vi "Auto - 副本.vi"() -> ()   [LabVIEW 2020]
uses:
  <vilib>/Utility/miscctls.llb/LVRowAndColumnTypeDef.ctl
  Global_Variable/A131258.vi
  Global_Variable/Global.vi
  Database/Global1.vi
  <vilib>/addons/database/Connection.llb/DB Tools Open Connec (String).vi
  <vilib>/addons/database/Connection.llb/Conn Execute.vi
  <vilib>/addons/database/Recordset.llb/Rec Fetch Recordset Data (R).vi
  Libraries/S7/S7.lvlib
  <vilib>/addons/database/NI_Database_API.lvlib
panel:
  out "左工位":cluster{dbl[], dbl[]}[](graph)
  in  "判定结果 2":bool[][](array[boolean])=[[TRUE]]
  out "STEP 4":string
  out "STEP 3":string
  in  "STEP 2":string
  out "右code 2":string
  in  "Initialize 7":bool
  in  "Initialize 6":bool
  out "初始化 2":bool[](array[boolean])
  out "左code":string
  out "右工位":cluster{dbl[], dbl[]}[](graph)
  in  "Initialize 4":bool
  in  "Initialize 2":bool
  out "初始化":bool[](array[boolean])
  in  "判定结果":bool[][](array[boolean])=[[TRUE]]
  in  "STEP":string
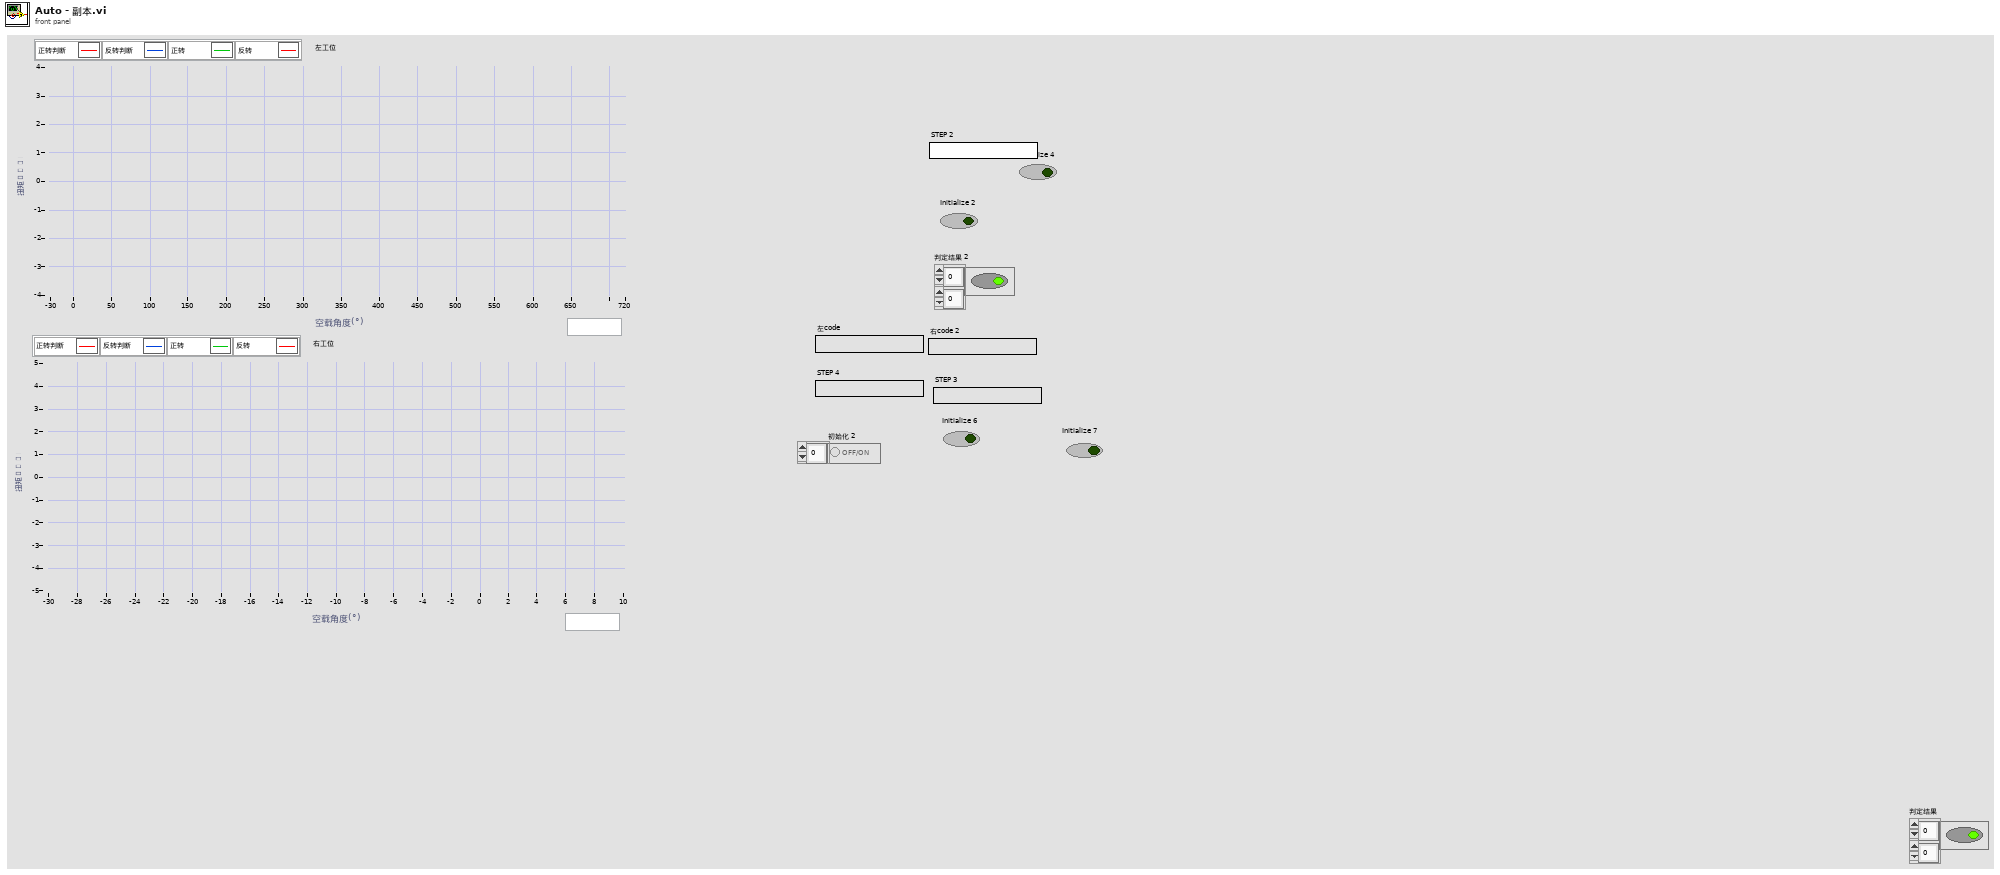
[diagram p1: front panel]
types:
  T1 = enum32{"Invalid", "Standard", "Closed", "Hidden", "Minimized", "Maximized"}
  T2 = typedef "LVRowAndColumnTypeDef.ctl" = cluster{"Row":i32, "Column":i32}
  T3 = typedef "lveventtype.ctl" = enum32{"Null", "Timeout", "Annotation Menu Selection", "Annotation Menu Selection?", "App Instance Close", "App Instance Close?", "Autoscale Range Change", "Bookmark Info Change", "Cell Edit", "Cell Edit?", "Cursor Grab", "Cursor Grab?", "Cursor Menu Selection", "Cursor Menu Selection?", "Cursor Move", "Cursor Release", "Data Change", "Direction Change", "Display State Change", "Drag Ended", "Drag Enter", "Drag Leave", "Drag Over", "Drag Source Update", "Drag Starting", "Drag Starting?", "Drop", "Exec State Change", "Key Down", "Key Down?", "Key Repeat", "Key Repeat?", "Key Up", "Listbox Double Click", "Menu Activation?", "Menu Selection (App)", "Menu Selection? (App)", "Menu Selection (User)", "Mouse Down", "Mouse Down?", "Mouse Enter", "Mouse Leave", "Mouse Move", "Mouse Up", "Mouse Wheel", "NI Security User Change (App)", "Pane Size", "Panel Close", "Panel Close?", "Panel Resize", "Plot Attribute Change", "Scale Range Change", "Shortcut Menu Activation?", "Shortcut Menu Selection (App)", "Shortcut Menu Selection? (App)", "Shortcut Menu Selection (User)", "Tree Double Click", "Tree Drag", "Tree Drag?", "Tree Drop", "Tree Drop?", "Tree Item Close", "Tree Item Close?", "Tree Item Open", "Tree Item Open?", "User Event", "Value Change"}
  T4 = typedef "LVPoint32TypeDef.ctl" = cluster{"Horizontal":i32, "Vertical":i32}
  T5 = cluster{"扭矩判定":cluster{"单位":string, "下限":dbl, "上限":dbl}, "正转扭矩最大值":cluster{"单位":string, "下限":dbl, "上限":dbl}, "正转扭矩最小值":cluster{"单位":string, "下限":dbl, "上限":dbl}, "正转扭矩波动值":cluster{"单位":string, "下限":dbl, "上限":dbl}, "正转平均扭矩值":cluster{"单位":string, "下限":dbl, "上限":dbl}, "反转扭矩最大值":cluster{"单位":string, "下限":dbl, "上限":dbl}, "反转扭矩最小值":cluster{"单位":string, "下限":dbl, "上限":dbl}, "反转扭矩波动值":cluster{"单位":string, "下限":dbl, "上限":dbl}, "反转扭矩平均值":cluster{"单位":string, "下限":dbl, "上限":dbl}, "正/逆转平均扭矩差":cluster{"单位":string, "下限":dbl, "上限":dbl}}
  T6 = cluster{"正向判定X值":cluster{"单位":string, "下限":dbl, "上限":dbl}, "正向判定Y值":cluster{"单位":string, "下限":dbl, "上限":dbl}, "逆向判定X值":cluster{"单位":string, "下限":dbl, "上限":dbl}, "逆向判定Y值":cluster{"单位":string, "下限":dbl, "上限":dbl}}
  T7 = cluster{"左平均扭矩":cluster{"正转":dbl, "反转":dbl}, "左矩波动":cluster{"正转":dbl, "反转":dbl}, "左空载":cluster{"正转":dbl, "反转":dbl}, "右平均扭矩":cluster{"正转":dbl, "反转":dbl}, "右扭矩波动":cluster{"正转":dbl, "反转":dbl}, "右空载":cluster{"正转":dbl, "反转":dbl}, "扭矩对称":cluster{"左":dbl, "右":dbl}, "左零点漂移":cluster{"正":dbl, "反":dbl}, "右零点漂移":cluster{"正":dbl, "反":dbl}}
  T8 = typedef "NI_Database_API.lvlib/Conn ObjectReference.ctl" = refnum<k1>
  T9 = typedef "NI_Database_API.lvlib/Rec ObjectReference.ctl" = refnum<k1>
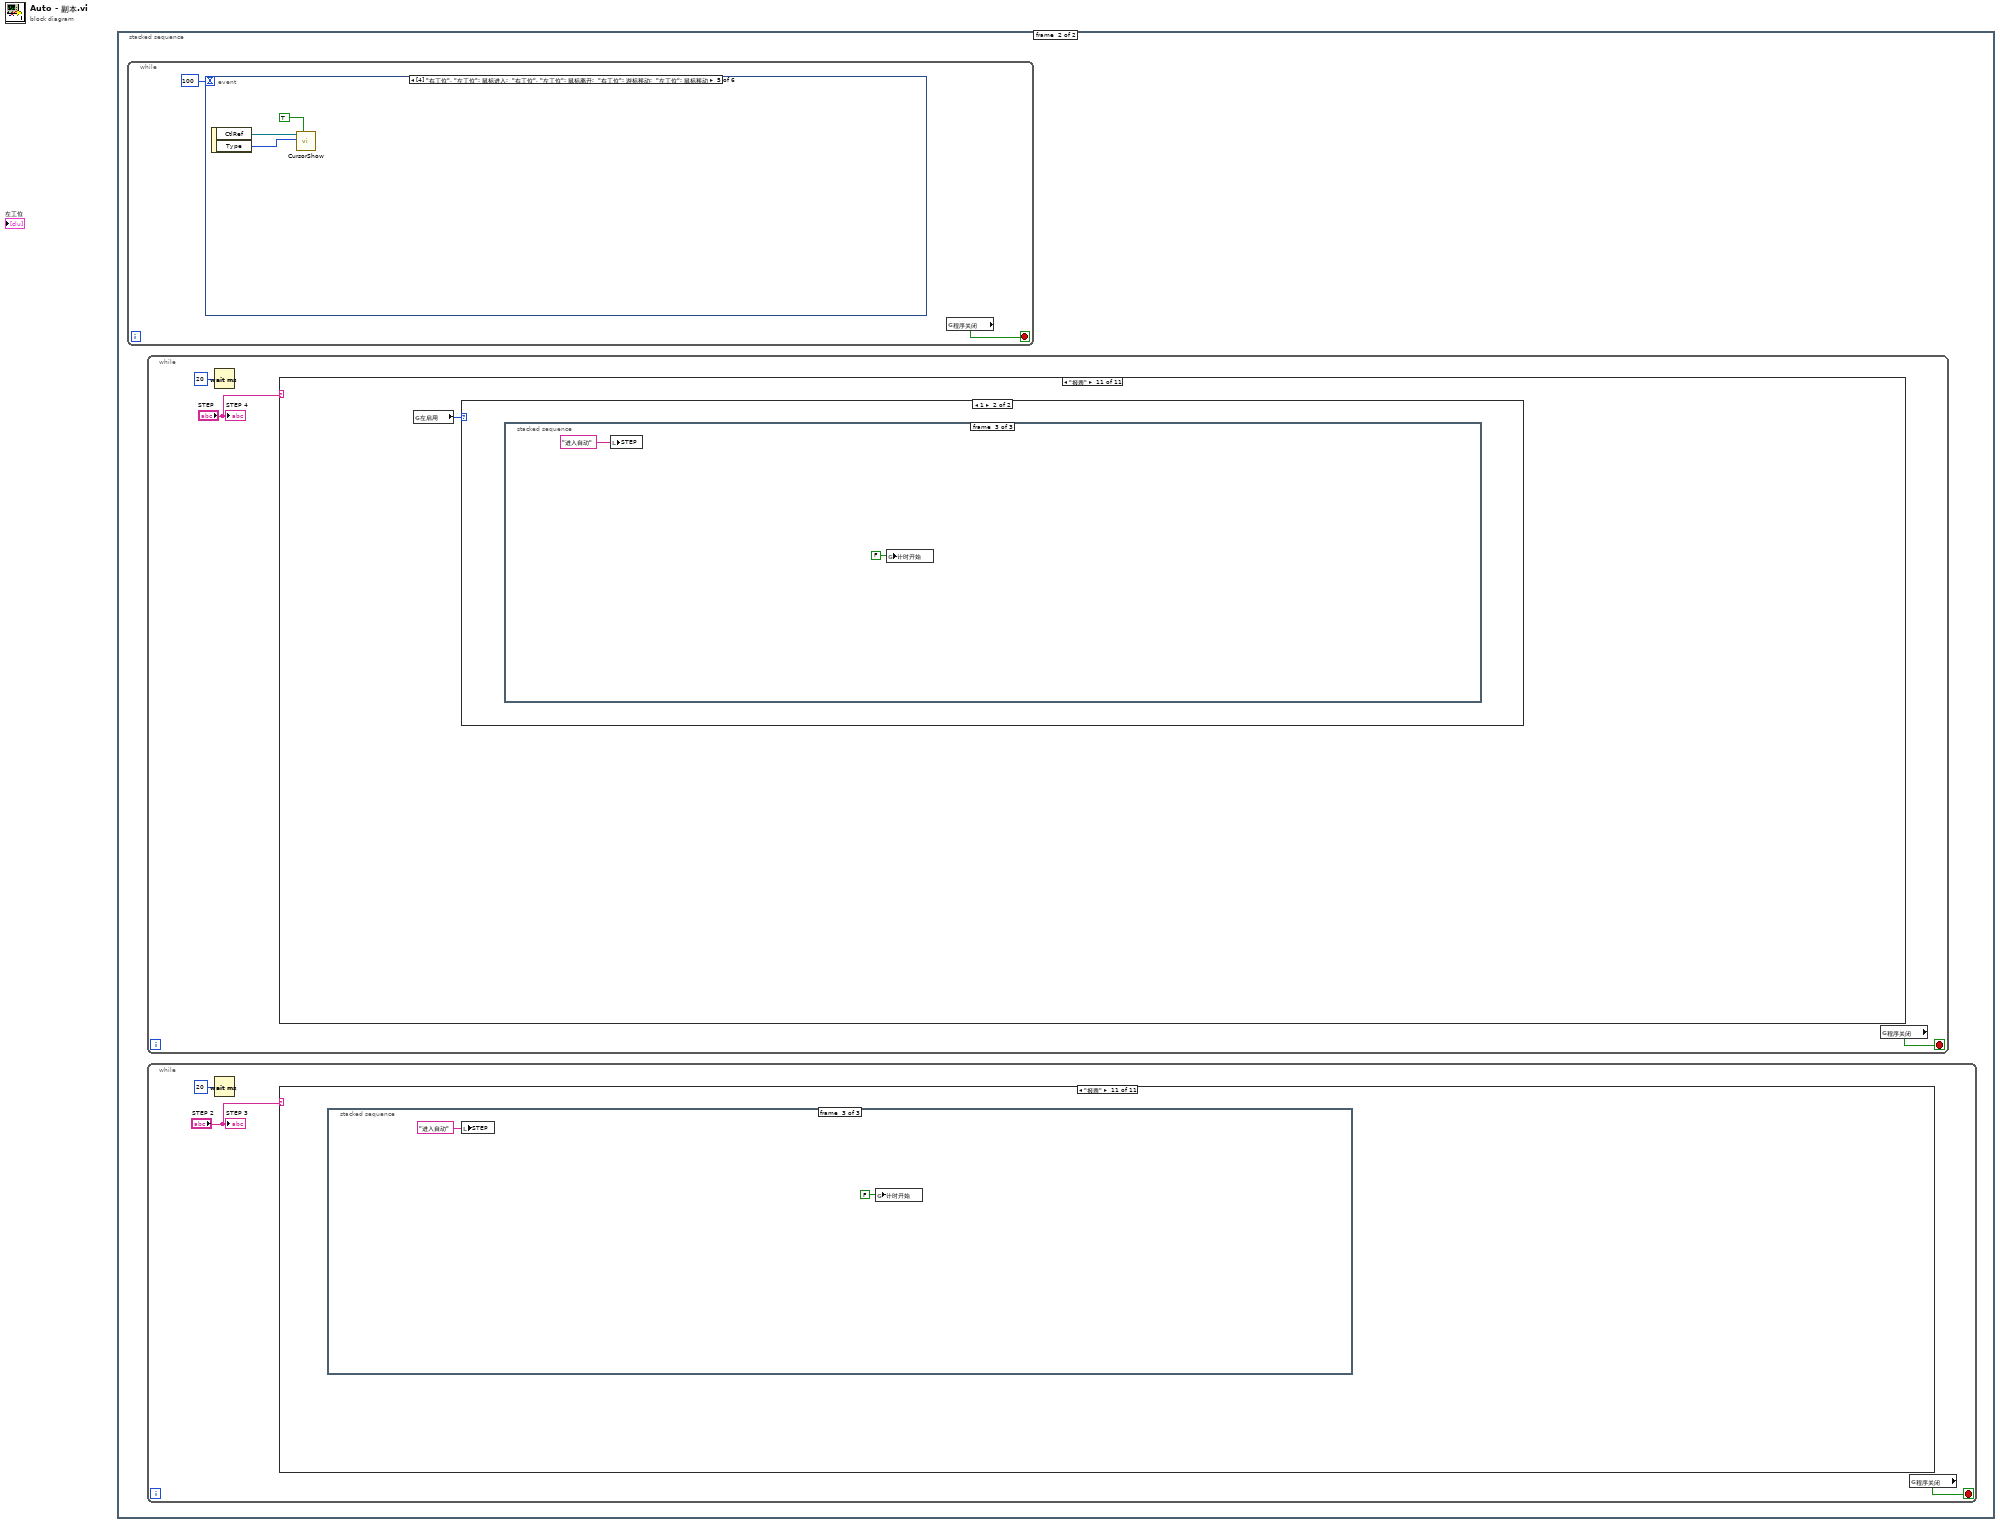
[diagram p0: block diagram]
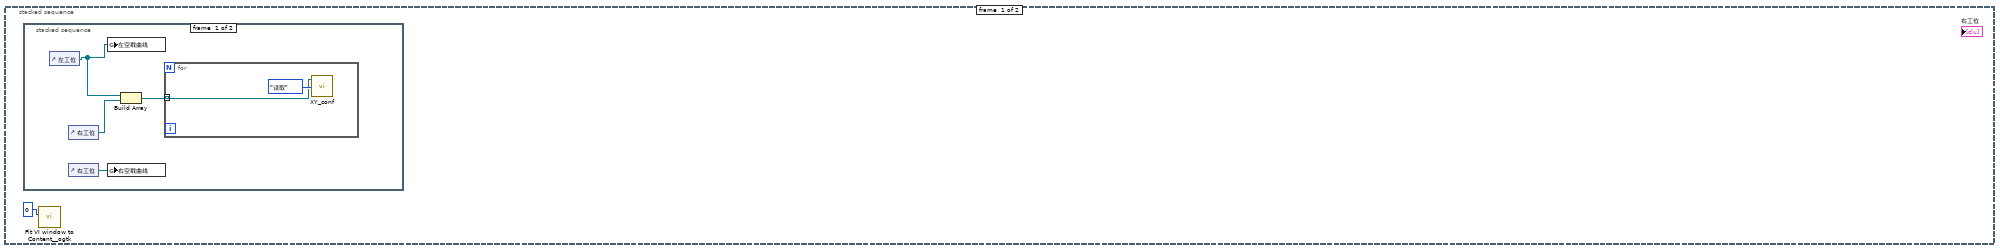
[diagram p2: hidden frame]
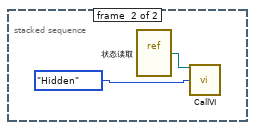
[diagram p3: hidden frame]
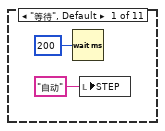
[diagram p4: hidden frame]
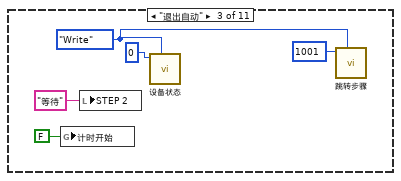
[diagram p6: hidden frame]
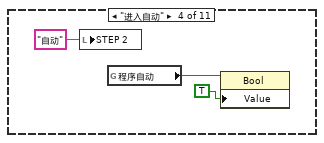
[diagram p7: hidden frame]
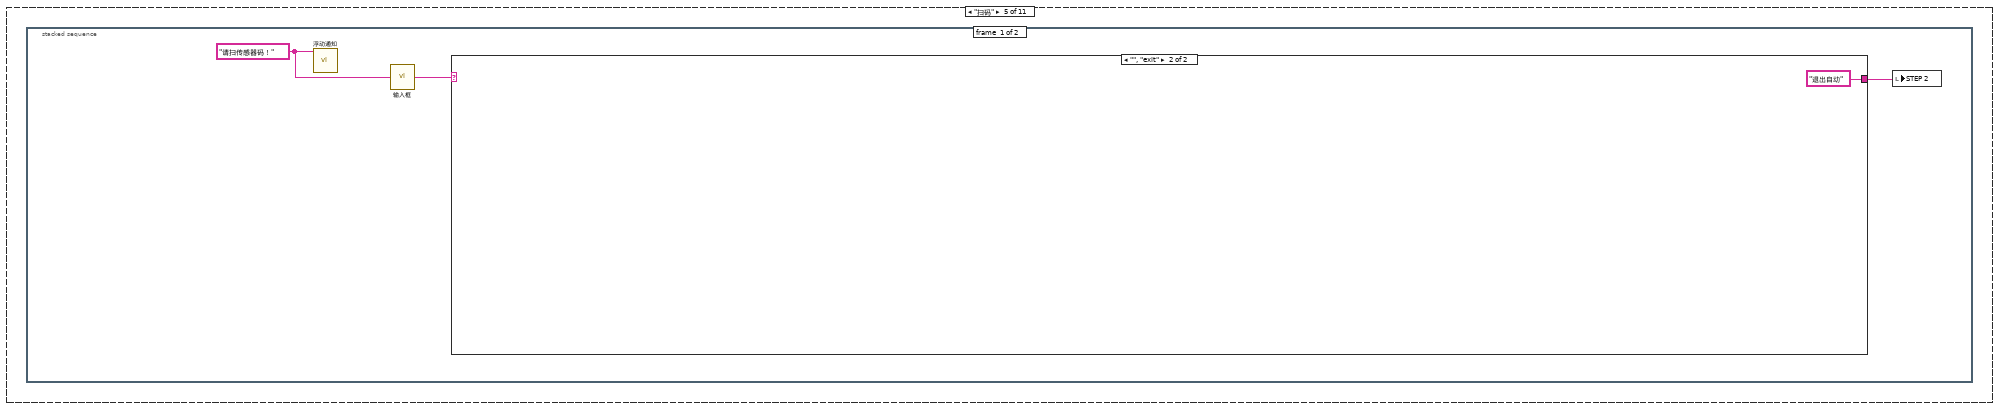
[diagram p8: hidden frame]
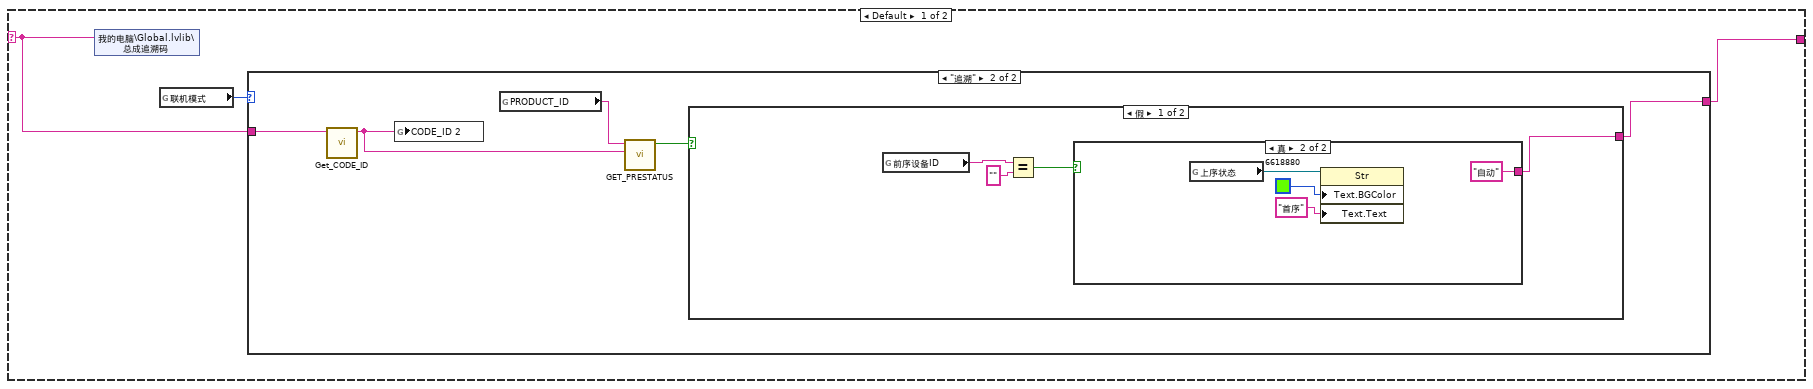
[diagram p9: hidden frame]
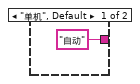
[diagram p10: hidden frame]
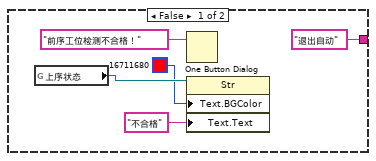
[diagram p11: hidden frame]
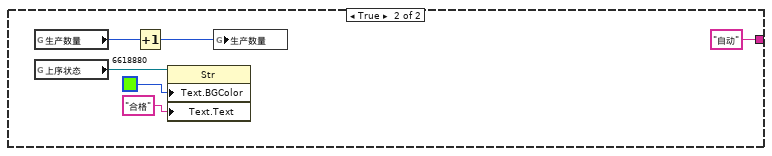
[diagram p12: hidden frame]
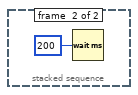
[diagram p13: hidden frame]
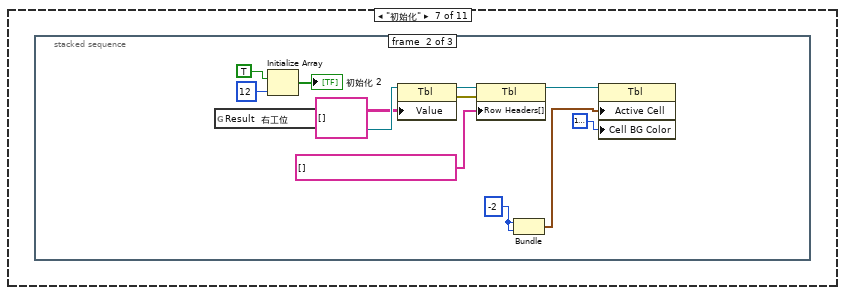
[diagram p15: hidden frame]
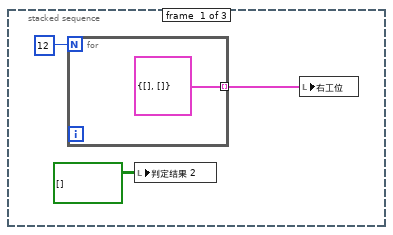
[diagram p16: hidden frame]
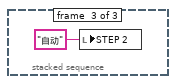
[diagram p17: hidden frame]
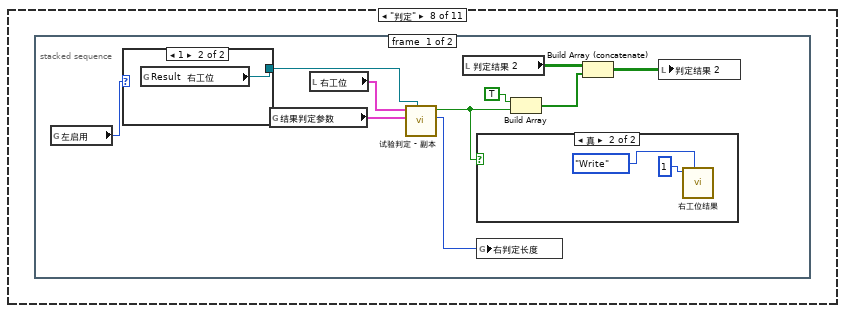
[diagram p18: hidden frame]
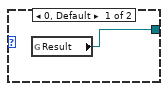
[diagram p19: hidden frame]
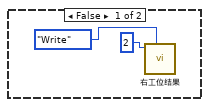
[diagram p20: hidden frame]
diagram:
  n1 = stacked-sequence {
    frame #0 {
      n2 = stacked-sequence {
        frame #0 {
          n3 = control-ref of="左工位"() -> (w2:refnum<vi>)
          n4 = control-ref of="右工位"() -> (w4:refnum<vi>)
          n5 = control-ref of="右工位"() -> (w5:refnum<vi>)
          n6 = global write "A131258.vi" "左空载曲线"(w2) -> ()
          n7 = global write "A131258.vi" "右空载曲线"(w5) -> ()
          n8 = Build Array(w2, w4) -> (w3:refnum<vi>[])
          n9 = for {
            tunnel: w3 -> [w6] mode=indexing
            n10 = call "XY_conf.vi"("方式"=enum16{"写入", "读取"}."读取", "XY图引用"=w6) -> ()  [unwired: 3 in, 1 out]
          }
        }
        frame #1 {
          n11 = vi-ref "状态读取.vi"() -> (w9:refnum<vi>)
          n12 = call "CallVI.vi"("VI引用"=w9, "状态"=T1."Hidden") -> ()  [unwired: 11 in, 3 out]
        }
      }
      n13 = call <userlib>:"Fit VI window to Content__ogtk.vi"("border spacing (2 px)"=0) -> ()  [unwired: 5 in, 2 out]
    }
    frame #1 {
      n14 = while {
        stop <- w748 stop-if-true
        n15 = event shown="[4] \"右工位\", \"左工位\": 鼠标进入;  \"右工位\", \"左工位\": 鼠标离开;  \"右工位\": 游标移动;  \"左工位\": 鼠标移动" {
          selector: _ -> [_ _ _ _ _ _]
          dyn-events: _ -> [_ _ _ _ _ _]
          timeout: 100 -> [_ _ _ _ _ _]
          event Timeout {
            n16 = event-data() -> ()  [unwired: 1 in, 3 out]
            n17 = call "Obtain Broadcast Events for Registration.vi"() -> ("Already running?"=w750:bool)  [unwired: 9 in, 2 out]
            n18 = case shown="真" w750 {
              frame False {
                n19 = local write "STEP"("手动" ("STEP")) -> ()
              }
              frame True {
                n20 = call "错误代码.vi"() -> ("Status_Read"=w752:u32)  [unwired: 11 in]
                n21 = case shown="0" w752 {
                  frame 0 {
                    n22 = global read "Global.vi" "报警图标"() -> (w763:refnum<vi>)
                    n23 = property class="Bool"(reference=w763, "Visible"=FALSE ("可见")) -> ()  [unwired: 1 in, 2 out]
                  }
                  frame 1, Default {
                    n24 = global read "Global.vi" "报警图标"() -> (w766:refnum<vi>)
                    n25 = property class="Bool"(reference=w766, "Visible"=TRUE ("可见")) -> ()  [unwired: 1 in, 2 out]
                  }
                }
                n26 = feedback #1() -> (w762:u32)  [unwired: 1 in]
                n27 = feedback-in #1(w752) -> ()
                n28 = Greater Or Equal?(x=w752, y=i16 5000) -> (x >= y?=w760:bool)
                n29 = Less?(x=w752, y=i16 5200) -> (x < y?=w761:bool)
                n30 = Equal?(x=w752, y=w762) -> (x = y?=w759:bool)
                n31 = global read "Global.vi" "报警图标"() -> (w754:refnum<vi>)
                n32 = And(x=w760, y=w761) -> (x .and. y?=w753:bool)
                n33 = property class="Bool"(reference=w754, "Value"=w753) -> ()  [unwired: 1 in, 2 out]
                n34 = Bundle By Name(cluster=errorcluster {"status"=FALSE, "code"=0, "source"=""} ("错误常量"), "status"=w753, "code"=w752) -> (w758:errorcluster)
                n35 = case shown="假" w759 {
                  tunnel: w758 -> [w767 _]
                  frame False {
                    n36 = call "报警处理.vi"("错误常量"=w767) -> ()  [unwired: 9 in, 2 out]
                  }
                  frame True {
                  }
                }
              }
            }
          }
          event Menu Selection (User) {
            n37 = event-data() -> ("ItemTag"=w768:string)  [unwired: 1 in, 2 out]
            n38 = case shown="\"真\"" w768 {
              frame "假", Default {
              }
              frame "真" {
              }
            }
          }
          event "右工位", "左工位": Scale Range Change {
            n39 = event-data() -> ("CtlRef"=w769:refnum<vi>)  [unwired: 1 in]
            n40 = call "XY_conf.vi"("方式"=enum16{"写入", "读取"}."写入", "XY图引用"=w769) -> ()  [unwired: 3 in, 1 out]
          }
          event Panel Close {
            n41 = event-data() -> ()  [unwired: 1 in, 4 out]
            n42 = global write "Global.vi" "程序关闭"(TRUE ("程序关闭")) -> ()
          }
          event "右工位", "左工位": Mouse Enter; "右工位", "左工位": Mouse Leave; "右工位": Cursor Move; "左工位": Mouse Move {
            n43 = event-data() -> ("CtlRef"=w774:refnum<vi>, "Type"=w773:T3)  [unwired: 1 in]
            n44 = call "CursorShow.vi"("nameShow"=TRUE, "Type"=w773, "Graph"=w774) -> ()  [unwired: 7 in, 2 out]
          }
          event "右工位", "左工位": Mouse Down {
            n45 = event-data() -> ("CtlRef"=w779:refnum<vi>, "Coords"=w778:T4, "Type"=w777:T3)  [unwired: 1 in]
            n46 = invoke class="XYGraph (严格)" method="Map Coords To XY"(reference=w779, "Coords"=w778) -> (reference out=w776:refnum<vi>, "XY"=w775:cluster{"X":dbl, "Y":dbl})  [unwired: 5 in, 5 out]
            n47 = call "CursorShow.vi"("游标.游标位置"=w775, "Type"=w777, "Graph"=w776) -> ()  [unwired: 7 in, 2 out]
          }
        }
        n48 = global read "Global.vi" "程序关闭"() -> (w748:bool)
      }
      n49 = while {
        stop <- w374 stop-if-true
        n50 = Wait (ms)(milliseconds to wait=u32 20 ("等待时间（毫秒）")) -> ()  [unwired: 1 out]
        n51 = case shown="\"报表\"" "STEP" {
          frame "等待", Default {
            n52 = Wait (ms)(milliseconds to wait=u32 200 ("等待时间（毫秒）")) -> ()  [unwired: 1 out]
            n53 = local write "STEP"("自动" ("STEP")) -> ()
          }
          frame "手动" {
          }
          frame "退出自动" {
            w378 = enum16{"Read", "Write"}."Write" ("枚举")
            n54 = global write "Global.vi" "计时开始"(FALSE ("计时开始")) -> ()
            n55 = local write "STEP"("等待" ("STEP")) -> ()
            n56 = call "设备状态.vi"("枚举"=w378, "Status_Write"=i16 0) -> ()  [unwired: 9 in, 1 out]
            n57 = call "跳转步骤.vi"("枚举"=w378, "Status_Write"=i16 1001) -> ()  [unwired: 9 in, 1 out]
          }
          frame "进入自动" {
            n58 = local write "STEP"("自动" ("STEP")) -> ()
            n59 = global read "Global.vi" "程序自动"() -> (w383:refnum<vi>)
            n60 = property class="Bool"(reference=w383, "Value"=TRUE) -> ()  [unwired: 1 in, 2 out]
          }
          frame "扫码" {
            n61 = stacked-sequence {
              frame #0 {
                w386 = "请扫传感器码！" ("提示信息")
                n62 = call "浮动通知.vi"("通知内容"=w386) -> ()  [unwired: 11 in]
                n63 = call "输入框.vi"("提示信息"=w386) -> ("条形码输出"=w387:string)
                n64 = case shown="\"\", \"exit\"" w387 {
                  selector: w387 -> [w388 _]
                  tunnel: [w390 "退出自动" ("State(s) in Front (\"\")")] -> w385
                  frame Default {
                    n65 = shared-variable "我的电脑\\Global.lvlib\\工位追溯码"(w388) -> ()  [unwired: 1 in, 1 out]
                    n66 = global read "Global1.vi" "联机模式"() -> (w389:enum16{"单机", "追溯"})
                    n67 = case shown="\"追溯\"" w389 {
                      tunnel: ["自动" ("State(s) in Front (\"\")") w396] -> w390
                      tunnel: w388 -> [_ w395]
                      frame "单机", Default {
                      }
                      frame "追溯" {
                        n68 = call "Get_CODE_ID.vi"("CODE_MAIN"=w395) -> ("CODE_ID"=w392:string)  [unwired: 10 in]
                        n69 = global write "追溯Global.vi" "CODE_ID"(w392) -> ()
                        n70 = global read "追溯Global.vi" "PRODUCT_ID"() -> (w394:string)
                        n71 = call "GET_PRESTATUS.vi"("CODE_ID"=w392, "PRODUCT_ID"=w394) -> ("OK?"=w393:bool)  [unwired: 8 in, 1 out]
                        n72 = case shown="真" w393 {
                          tunnel: [w400 "自动" ("State(s) in Front (\"\")")] -> w396
                          frame False {
                            n73 = global read "追溯Global.vi" "前序设备ID"() -> (w399:string)
                            n74 = Equal?(x=w399, y="") -> (x = y?=w398:bool)
                            n75 = case shown="真" w398 {
                              tunnel: ["退出自动" ("State(s) in Front (\"\")") "自动" ("State(s) in Front (\"\")")] -> w400
                              frame False {
                                n76 = global read "Global.vi" "上序状态"() -> (w403:refnum<vi>)
                                n77 = One Button Dialog(message="前序工位检测不合格！" ("消息")) -> ()  [unwired: 1 in, 1 out]
                                n78 = property class="Str"(reference=w403, "Text.BGColor"=u32 16711680 ("文本.文本颜色:背景色"), "Text.Text"="不合格" ("文本.文本")) -> ()  [unwired: 1 in, 2 out]
                              }
                              frame True {
                                n79 = global read "Global.vi" "上序状态"() -> (w408:refnum<vi>)
                                n80 = property class="Str"(reference=w408, "Text.BGColor"=u32 6618880 ("文本.文本颜色:背景色"), "Text.Text"="首序" ("文本.文本")) -> ()  [unwired: 1 in, 2 out]
                              }
                            }
                          }
                          frame True {
                            n81 = global read "Global.vi" "生产数量"() -> (w413:i32)
                            n82 = global read "Global.vi" "上序状态"() -> (w412:refnum<vi>)
                            n83 = Increment(x=w413) -> (x+1=w414:i32)
                            n84 = property class="Str"(reference=w412, "Text.BGColor"=u32 6618880 ("文本.文本颜色:背景色"), "Text.Text"="合格" ("文本.文本")) -> ()  [unwired: 1 in, 2 out]
                            n85 = global write "Global.vi" "生产数量"(w414) -> ()
                          }
                        }
                      }
                    }
                  }
                  frame "", "exit" {
                  }
                }
                n86 = local write "STEP"(w385) -> ()
              }
              frame #1 {
                n87 = Wait (ms)(milliseconds to wait=u32 200 ("等待时间（毫秒）")) -> ()  [unwired: 1 out]
              }
            }
          }
          frame "工位判断" {
          }
          frame "初始化" {
            n88 = stacked-sequence {
              frame #0 {
                n89 = global write "Global.vi" "IO_Stop"(TRUE ("IO_Stop")) -> ()
                n90 = global write "Global.vi" "计时开始"(TRUE ("计时开始")) -> ()
                n91 = local write "判定结果"(bool[][] [] ("判定结果")) -> ()
              }
              frame #1 {
                n92 = for {
                  N: 12 -> [_]
                  tunnel: [cluster{dbl[], dbl[]} {[], []}] -> w421 mode=indexing
                }
                n93 = local write "左工位"(w421) -> ()
              }
              frame #2 {
                w424 = -2 ("维数大小")
                n94 = global read "Global.vi" "Result"() -> (w433:refnum<vi>)
                n95 = Initialize Array(TRUE, 12 ("维数大小")) -> (→"初始化":bool[])
                n96 = property class="Tbl"(reference=w433, "Value"=string[][] []) -> (reference out=w434:refnum<vi>, error out=w435:errorcluster)  [unwired: 1 in]
                n97 = property class="Tbl"(reference=w434, error in=w435, "Row Headers[]"=string[] [] ("列首字符串[]")) -> (reference out=w427:refnum<vi>)  [unwired: 1 out]
                n98 = Bundle("维数大小"=w424, "维数大小"=w424) -> (w425:cluster{"维数大小":i32, "维数大小":i32})  [unwired: 1 in]
                n99 = property class="Tbl"(reference=w427, "Active Cell"=w425, "Cell BG Color"=u32 16777216 ("活动单元格:单元格背景色")) -> ()  [unwired: 1 in, 2 out]
              }
              frame #3 {
                n100 = local write "STEP"("自动" ("STEP")) -> ()
              }
            }
          }
          frame "判定" {
            n101 = stacked-sequence {
              frame #0 {
                n102 = global read "A131258.vi" "结果判定参数"() -> (w438:T5)
                n103 = global read "Global.vi" "Result"() -> (w440:refnum<vi>)
                n104 = local read "左工位"() -> (w439:cluster{dbl[], dbl[]}[])
                n105 = call "试验判定.vi"("Result"=w440, "判定参数"=w438, "XY曲线"=w439) -> ("判定项长度"=w437:i32, "OK？"=w441:bool)  [unwired: 7 in]
                n106 = case shown="真" w441 {
                  frame False {
                    n107 = call "左工位结果.vi"("枚举"=enum16{"Read", "Write"}."Write", "Status_Write"=u16 2 ("左工位生产结果")) -> ()  [unwired: 9 in, 1 out]
                  }
                  frame True {
                    n108 = call "左工位结果.vi"("枚举"=enum16{"Read", "Write"}."Write", "Status_Write"=u16 1 ("左工位生产结果")) -> ()  [unwired: 9 in, 1 out]
                  }
                }
                n109 = global write "判定参数.vi" "左判定长度"(w437) -> ()
                n110 = Build Array(TRUE ("元素"), w441) -> (w444:bool[])
                n111 = local read "判定结果"() -> (w445:bool[][])
                n112 = Build Array(w444) -> (w443:bool[][])
                n113 = Build Array (concatenate)(w445, w443) -> (w446:bool[][])
                n114 = local write "判定结果"(w446) -> ()
              }
              frame #1 {
                n115 = local write "STEP"("报表" ("STEP")) -> ()
              }
            }
          }
          frame "自动" {
            n116 = global read "Global.vi" "跳转"() -> (w452:i16)
            n117 = global read "Global.vi" "左状态"() -> (w453:i16)
            n118 = case shown="1003" w452 {
              frame 0, Default {
              }
              frame 1000 {
                n119 = stacked-sequence {
                  frame #0 {
                    w454 = "" ("文本.文本")
                    n120 = Wait (ms)(milliseconds to wait=u32 200 ("等待时间（毫秒）")) -> ()  [unwired: 1 out]
                    n121 = shared-variable "我的电脑\\Global.lvlib\\传感器码-左"(w454) -> ()  [unwired: 1 in, 1 out]
                    n122 = shared-variable "我的电脑\\Global.lvlib\\传感器码-右"(w454) -> ()  [unwired: 1 in, 1 out]
                    n123 = call "跳转步骤.vi"("枚举"=enum16{"Read", "Write"}."Write", "Status_Write"=u16 1001 ("跳转步骤")) -> ()  [unwired: 9 in, 1 out]
                  }
                  frame #1 {
                    n124 = local write "STEP"("扫码" ("STEP")) -> ()
                  }
                }
              }
              frame 1001 {
                n125 = stacked-sequence {
                  frame #0 {
                    n126 = Wait (ms)(milliseconds to wait=u32 100 ("等待时间（毫秒）")) -> ()  [unwired: 1 out]
                  }
                  frame #1 {
                    n127 = global read "Global.vi" "左在位"() -> (w461:i16)
                    n128 = global read "Global.vi" "右在位"() -> (w460:i16)
                    n129 = case shown="1" w461 {
                      frame 0, Default {
                      }
                      frame 1 {
                        w466 = enum16{"Read", "Write"}."Write" ("枚举")
                        n130 = call "左工位在位.vi"("枚举"=w466, "Status_Write"=u16 0 ("左工位工件在位")) -> ()  [unwired: 9 in, 1 out]
                        n131 = call "左工位状态.vi"("枚举"=w466, "Status_Write"=u16 1001 ("左工位状态")) -> ()  [unwired: 9 in, 1 out]
                      }
                    }
                    n132 = case shown="1" w460 {
                      frame 0, Default {
                      }
                      frame 1 {
                        w462 = enum16{"Read", "Write"}."Write" ("枚举")
                        n133 = call "右工位在位.vi"("枚举"=w462, "Status_Write"=u16 0 ("右工位工件在位")) -> ()  [unwired: 9 in, 1 out]
                        n134 = call "右工位状态.vi"("枚举"=w462, "Status_Write"=u16 1001 ("左工位状态")) -> ()  [unwired: 9 in, 1 out]
                      }
                    }
                  }
                  frame #2 {
                    n135 = local write "STEP 2"("自动" ("STEP")) -> ()
                    n136 = local write "STEP"("自动" ("STEP")) -> ()
                  }
                }
              }
              frame 1002 {
                # "SELECT CODE_ID FROM CODE  WHERE CODE_SENSOR = '"
                n137 = stacked-sequence {
                  frame #0 {
                    n138 = Wait (ms)(milliseconds to wait=u32 200 ("等待时间（毫秒）")) -> ()  [unwired: 1 out]
                    n139 = call "跳转步骤.vi"("枚举"=enum16{"Read", "Write"}."Write", "Status_Write"=u16 1003 ("跳转步骤")) -> ()  [unwired: 9 in, 1 out]
                  }
                  frame #1 {
                    n140 = local write "STEP 2"("扫码" ("STEP")) -> ()
                  }
                }
              }
              frame 1003 {
                n141 = stacked-sequence {
                  frame #0 {
                    n142 = Wait (ms)(milliseconds to wait=u32 100 ("等待时间（毫秒）")) -> ()  [unwired: 1 out]
                  }
                  frame #1 {
                    n143 = global read "Global.vi" "左在位"() -> (w476:i16)
                    n144 = global read "Global.vi" "右在位"() -> (w475:i16)
                    n145 = case shown="1" w476 {
                      frame 0, Default {
                      }
                      frame 1 {
                        w480 = enum16{"Read", "Write"}."Write" ("枚举")
                        n146 = call "左工位在位.vi"("枚举"=w480, "Status_Write"=u16 0 ("左工位工件在位")) -> ()  [unwired: 9 in, 1 out]
                        n147 = call "左工位状态.vi"("枚举"=w480, "Status_Write"=u16 1002 ("左工位状态")) -> ()  [unwired: 9 in, 1 out]
                      }
                    }
                    n148 = case shown="1" w475 {
                      frame 0, Default {
                      }
                      frame 1 {
                        w477 = enum16{"Read", "Write"}."Write" ("枚举")
                        n149 = call "右工位在位.vi"("枚举"=w477, "Status_Write"=u16 0 ("右工位工件在位")) -> ()  [unwired: 9 in, 1 out]
                        n150 = call "右工位状态.vi"("枚举"=w477, "Status_Write"=u16 1002 ("左工位状态")) -> ()  [unwired: 9 in, 1 out]
                      }
                    }
                  }
                  frame #2 {
                    w483 = "自动" ("STEP")
                    n151 = local write "STEP"(w483) -> ()
                    n152 = local write "STEP 2"(w483) -> ()
                  }
                }
              }
            }
            n153 = case shown="1002" w453 {
              frame 0, Default {
              }
              frame 1 {
              }
              frame 3 {
                n154 = stacked-sequence {
                  frame #0 {
                    n155 = call "左工位结果.vi"("枚举"=enum16{"Read", "Write"}."Write", "Status_Write"=i16 0) -> ()  [unwired: 9 in, 1 out]
                    n156 = local write "判定结果"(bool[][] [] ("判定结果")) -> ()
                  }
                  frame #1 {
                    n157 = global read "Global.vi" "空载速度(°/s) 2"() -> (w487:sgl)
                    n158 = Multiply(x=w487, y=sgl 6.0) -> (x*y=w488:sgl)
                    n159 = global write "Global.vi" "空载速度(°/s)"(w488) -> ()
                  }
                }
              }
              frame 200 {
                n160 = stacked-sequence {
                  frame #0 {
                    w490 = TRUE ("Initialize 2")
                    n161 = local write "Initialize 2"(w490) -> ()
                    n162 = local write "Initialize 4"(w490) -> ()
                    n163 = call "左工位结果.vi"("枚举"=enum16{"Read", "Write"}."Write", "Status_Write"=u16 0 ("左工位生产结果")) -> ()  [unwired: 9 in, 1 out]
                  }
                  frame #1 {
                    n164 = local read "左工位"() -> (w493:cluster{dbl[], dbl[]}[])
                    n165 = for {
                      tunnel: [w496] -> w494 mode=indexing
                      tunnel: w493 -> [w495] mode=indexing
                      i -> [w497]
                      n166 = case shown="1" w497 {
                        tunnel: [w498 w499 w507] -> w496
                        tunnel: w495 -> [w498 _ _]
                        frame Default {
                        }
                        frame 0 {
                          n167 = global read "A131258.vi" "判定框参数"() -> (w504:T6)
                          n168 = Unbundle By Name(w504) -> ("正向判定X值.下限"=w503:dbl, "正向判定X值.上限"=w502:dbl, "正向判定Y值.下限"=w501:dbl, "正向判定Y值.上限"=w500:dbl)
                          n169 = Build Array(w502, w502, w503, w503, w502) -> (w506:dbl[])
                          n170 = Build Array(w500, w501, w501, w500, w500) -> (w505:dbl[])
                          n171 = Bundle(w506, w505) -> (w499:cluster{dbl[], dbl[]})  [unwired: 1 in]
                        }
                        frame 1 {
                          n172 = global read "A131258.vi" "判定框参数"() -> (w512:T6)
                          n173 = Unbundle By Name(w512) -> ("逆向判定X值.下限"=w511:dbl, "逆向判定X值.上限"=w510:dbl, "逆向判定Y值.下限"=w509:dbl, "逆向判定Y值.上限"=w508:dbl)
                          n174 = Build Array(w510, w510, w511, w511, w510) -> (w514:dbl[])
                          n175 = Build Array(w508, w509, w509, w508, w508) -> (w513:dbl[])
                          n176 = Bundle(w514, w513) -> (w507:cluster{dbl[], dbl[]})  [unwired: 1 in]
                        }
                      }
                    }
                    n177 = local write "左工位"(w494) -> ()
                  }
                }
              }
              frame 500 {
                n178 = local read "左工位"() -> (w516:cluster{dbl[], dbl[]}[])
                n179 = for {
                  tunnel: w516 -> [w518] mode=indexing
                  tunnel: [w517] -> w515 mode=indexing
                  i -> [w519]
                  n180 = case shown="2" w519 {
                    tunnel: w518 -> [w520 w537]
                    tunnel: [w520 w528] -> w517
                    frame Default {
                    }
                    frame 2 {
                      n181 = local write "Initialize 2"(FALSE ("Initialize 2")) -> ()
                      n182 = global read "A131258.vi" "系数"() -> (w523:T7)
                      n183 = case shown="假" "Initialize 2" {
                        tunnel: [w550 0.0] -> w533
                        frame False {
                          n184 = global read "全局 1.vi" "工位2正向磨合开始时间"() -> (w554:u32)
                          n185 = Tick Count (ms)() -> (millisecond timer value=w553:u32)
                          n186 = Subtract(x=w553, y=w554) -> (x-y=w552:u32)
                          n187 = Divide(x=w552, y=u32 1000) -> (x/y=w550:dbl)
                          n188 = global write "全局 1.vi" "工位2正向磨合结束时间"(w550) -> ()
                        }
                        frame True {
                          n189 = Tick Count (ms)() -> (millisecond timer value=w555:u32)
                          n190 = global write "全局 1.vi" "工位2正向磨合开始时间"(w555) -> ()
                        }
                      }
                      n191 = global read "A131258.vi" "零点标定"() -> (w524:bool)
                      n192 = global read "全局1.vi" "左加载"() -> (w522:dbl)
                      n193 = case shown="假" w524 {
                        tunnel: [w539 w546] -> w521
                        tunnel: w523 -> [w545 w549]
                        tunnel: w522 -> [w544 w548]
                        frame False {
                          n194 = Unbundle By Name(w545) -> ("左零点漂移.正"=w543:dbl, "左空载.正转"=w540:dbl, "左零点漂移.正"=w538:dbl)
                          n195 = Multiply(x=w544, y=w543) -> (x*y=w541:dbl)
                          n196 = Subtract(x=w541, y=w540) -> (x-y=w542:dbl)
                          n197 = Subtract(x=w542, y=w538) -> (x-y=w539:dbl)
                        }
                        frame True {
                          n198 = Unbundle By Name(w549) -> ("左零点漂移.正"=w547:dbl)
                          n199 = Subtract(x=w548, y=w547) -> (x-y=w546:dbl)
                        }
                      }
                      n200 = Unbundle(w537) -> (w530:dbl[], w536:dbl[])
                      n201 = Build Array (concatenate)(w536, w521) -> (w527:dbl[])
                      n202 = global read "Global.vi" "空载速度(°/s)"() -> (w532:sgl)
                      n203 = Divide(x=w533, y=1.0) -> (x/y=w526:dbl)
                      n204 = Multiply(x=w532, y=w526) -> (x*y=w531:dbl)
                      n205 = Build Array (concatenate)(w530, w531) -> (w529:dbl[])
                      n206 = Bundle(w529, w527) -> (w528:cluster{dbl[], dbl[]})  [unwired: 1 in]
                    }
                  }
                }
                n207 = local write "左工位"(w515) -> ()
              }
              frame 600 {
                n208 = local read "左工位"() -> (w558:cluster{dbl[], dbl[]}[])
                n209 = for {
                  tunnel: w558 -> [w560] mode=indexing
                  tunnel: [w559] -> w557 mode=indexing
                  i -> [w561]
                  n210 = case shown="3" w561 {
                    tunnel: w560 -> [w562 w579]
                    tunnel: [w562 w570] -> w559
                    frame 0, Default {
                    }
                    frame 3 {
                      n211 = local write "Initialize 4"(FALSE ("Initialize 2")) -> ()
                      n212 = case shown="假" "Initialize 4" {
                        tunnel: [w592 w599] -> w576
                        frame False {
                          n213 = global read "全局 1.vi" "工位2逆向磨合开始时间"() -> (w598:u32)
                          n214 = Tick Count (ms)() -> (millisecond timer value=w597:u32)
                          n215 = Subtract(x=w597, y=w598) -> (x-y=w596:u32)
                          n216 = global read "全局 1.vi" "工位2正向磨合结束时间"() -> (w594:dbl)
                          n217 = Divide(x=w596, y=u32 1000) -> (x/y=w593:dbl)
                          n218 = Subtract(x=w594, y=w593) -> (x-y=w592:dbl)
                        }
                        frame True {
                          n219 = Tick Count (ms)() -> (millisecond timer value=w600:u32)
                          n220 = global write "全局 1.vi" "工位2逆向磨合开始时间"(w600) -> ()
                          n221 = global read "全局 1.vi" "工位2正向磨合结束时间"() -> (w599:dbl)
                        }
                      }
                      n222 = global read "全局1.vi" "左加载"() -> (w564:dbl)
                      n223 = global read "A131258.vi" "系数"() -> (w565:T7)
                      n224 = global read "A131258.vi" "零点标定"() -> (w566:bool)
                      n225 = Unbundle(w579) -> (w573:dbl[], w578:dbl[])
                      n226 = case shown="假" w566 {
                        tunnel: [w581 w588] -> w563
                        tunnel: w565 -> [w587 w591]
                        tunnel: w564 -> [w586 w590]
                        frame False {
                          n227 = Unbundle By Name(w587) -> ("左零点漂移.反"=w585:dbl, "左空载.反转"=w582:dbl, "左零点漂移.反"=w580:dbl)
                          n228 = Multiply(x=w586, y=w585) -> (x*y=w583:dbl)
                          n229 = Subtract(x=w583, y=w582) -> (x-y=w584:dbl)
                          n230 = Subtract(x=w584, y=w580) -> (x-y=w581:dbl)
                        }
                        frame True {
                          n231 = Unbundle By Name(w591) -> ("左零点漂移.反"=w589:dbl)
                          n232 = Add(x=w590, y=w589) -> (x+y=w588:dbl)
                        }
                      }
                      n233 = Build Array (concatenate)(w578, w563) -> (w571:dbl[])
                      n234 = global read "Global.vi" "空载速度(°/s)"() -> (w575:sgl)
                      n235 = Divide(x=w576, y=1.0) -> (x/y=w568:dbl)
                      n236 = Multiply(x=w575, y=w568) -> (x*y=w574:dbl)
                      n237 = Build Array (concatenate)(w573, w574) -> (w572:dbl[])
                      n238 = Bundle(w572, w571) -> (w570:cluster{dbl[], dbl[]})  [unwired: 1 in]
                    }
                  }
                }
                n239 = local write "左工位"(w557) -> ()
              }
              frame 680 {
                n240 = local write "STEP"("判定" ("STEP")) -> ()
              }
              frame 1001 {
                n241 = stacked-sequence {
                  frame #0 {
                    n242 = Wait (ms)(milliseconds to wait=u32 50 ("等待时间（毫秒）")) -> ()  [unwired: 1 out]
                    n243 = shared-variable "我的电脑\\Global.lvlib\\工位追溯码"() -> (w602:string)  [unwired: 1 in, 1 out]
                    n244 = shared-variable "我的电脑\\Global.lvlib\\传感器码-左"(w602) -> ()  [unwired: 1 in, 1 out]
                  }
                  frame #1 {
                    n245 = global read "Global1.vi" "联机模式"() -> (w604:enum16{"单机", "追溯"})
                    n246 = case shown="\"追溯\"" w604 {
                      selector: w604 -> [_ w614]
                      frame "单机", Default {
                      }
                      frame "追溯" {
                        n247 = shared-variable "我的电脑\\Global.lvlib\\传感器码-左"() -> (w605:string)  [unwired: 1 in, 1 out]
                        n248 = global read "追溯Global.vi" "PRODUCT_ID"() -> (w611:string)
                        n249 = Bundle("String"=w605, "PRODUCT_ID"=w611) -> (w610:cluster{"String":string, "PRODUCT_ID":string})  [unwired: 1 in]
                        n250 = call "GetSQLstring.vi"("联机模式"=w614) -> ("错误输出"=w612:errorcluster, "连接字符串"=w613:string)  [unwired: 9 in]
                        n251 = call-poly <vilib>:"DB Tools Open Connection.vi"("error in (no error)"=w612, "connection information"=w613) -> ("error out"=w608:errorcluster, "connection reference"=w609:T8)  [unwired: 6 in]
                        n252 = Build Array(w610) -> (w606:cluster{"String":string, "PRODUCT_ID":string}[])
                        n253 = for {
                          tunnel: w609 -> [w622]
                          shift-right: [w619] -> w607
                          shift-left: w608 -> [w621]
                          tunnel: w606 -> [w615] mode=indexing
                          n254 = call <vilib>:"DB Tools Insert Data.vi"("data"=w615, "error in (no error)"=w621, "columns"=string[] ["CODE_SENSOR", "PRODUCT_ID"], "table"="Code", "connection reference"=w622) -> ("error out"=w620:errorcluster, "connection reference out"=w618:T8)  [unwired: 5 in]
                          n255 = case shown="错误 .." w620 {
                            selector: w620 -> [w624 w626]
                            tunnel: [w624 w627] -> w619
                            tunnel: [w623 w625] -> _
                            tunnel: w618 -> [w623 w625]
                            frame No Error {
                            }
                            frame Error {
                              n256 = call <vilib>:"Clear Errors.vi"("error in (no error)"=w626) -> ("error out"=w627:errorcluster)  [unwired: 5 in, 1 out]
                            }
                          }
                        }
                        n257 = call <vilib>:"Simple Error Handler.vi"("error in (no error)"=w607) -> ()  [unwired: 4 in, 5 out]
                      }
                    }
                  }
                  frame #2 {
                    n258 = global read "Global1.vi" "联机模式"() -> (w628:enum16{"单机", "追溯"})
                    n259 = case shown="\"追溯\"" w628 {
                      selector: w628 -> [_ w649]
                      frame "单机", Default {
                      }
                      frame "追溯" {
                        w641 = "'"
                        n260 = shared-variable "我的电脑\\Global.lvlib\\传感器码-左"() -> (w629:string)  [unwired: 1 in, 1 out]
                        n261 = global read "追溯Global.vi" "PRODUCT_ID"() -> (w642:string)
                        n262 = call "GetSQLstring.vi"("联机模式"=w649) -> ("错误输出"=w647:errorcluster, "连接字符串"=w648:string)  [unwired: 9 in]
                        n263 = Concatenate Strings("SELECT CODE_ID FROM CODE  WHERE CODE_SENSOR = '" ("table"), w629, w641, " AND PRODUCT_ID='" ("字符串"), w642, w641) -> (w640:string)
                        n264 = call-poly <vilib>:"DB Tools Open Connection.vi"("error in (no error)"=w647, "connection information"=w648) -> ("error out"=w646:errorcluster, "connection reference"=w645:T8)  [unwired: 6 in]
                        n265 = call-poly <vilib>:"DB Tools Execute Query.vi"("error in (no error)"=w646, "SQL query"=w640, "connection reference"=w645) -> ("error out"=w639:errorcluster, "recordset reference"=w638:T9)  [unwired: 5 in]
                        n266 = call-poly <vilib>:"DB Tools Fetch Recordset Data.vi"("error in (no error)"=w639, "recordset reference"=w638) -> ("error out"=w637:errorcluster, "recordset data"=w636:variant[][])  [unwired: 3 in, 1 out]
                        n267 = Variant To Data(error in=w637, type=string[][] [], Variant=w636) -> (data=w634:string[][])  [unwired: 1 out]
                        n268 = Index Array(array=w634, index (row)=0 ("索引 (行)")) -> (element=w633:string[])  [unwired: 1 in]
                        n269 = Index Array(array=w633, index=0 ("索引")) -> (element=→"左code":string)
                      }
                    }
                  }
                  frame #3 {
                    n270 = Wait (ms)(milliseconds to wait=u32 50 ("等待时间（毫秒）")) -> ()  [unwired: 1 out]
                    n271 = call "左工位状态.vi"("枚举"=enum16{"Read", "Write"}."Write", "Status_Write"=u16 1003 ("左工位状态")) -> ()  [unwired: 9 in, 1 out]
                    n272 = for {
                      N: 12 -> [_]
                      tunnel: [cluster{dbl[], dbl[]} {[], []}] -> w656 mode=indexing
                    }
                    n273 = local write "左工位"(w656) -> ()
                    n274 = global read "Global.vi" "Result"() -> (w654:refnum<vi>)
                    n275 = property class="Tbl"(reference=w654, "Row Headers[]"=string[] [] ("行首字符串[]"), "Value"=string[][] [] ("值"), "Active Cell"=T2 {"Row"=-2, "Column"=-2} ("活动单元格:活动单元格"), "Cell BG Color"=u32 16777216 ("活动单元格:单元格背景色")) -> ()  [unwired: 1 in, 2 out]
                  }
                }
              }
              frame 1002 {
                n276 = stacked-sequence {
                  frame #0 {
                    n277 = Wait (ms)(milliseconds to wait=u32 100 ("等待时间（毫秒）")) -> ()  [unwired: 1 out]
                    n278 = shared-variable "我的电脑\\Global.lvlib\\总成追溯码"() -> (w661:string)  [unwired: 1 in, 1 out]
                    n279 = shared-variable "我的电脑\\Global.lvlib\\传感器码-左"(w661) -> ()  [unwired: 1 in, 1 out]
                  }
                  frame #1 {
                    n280 = global read "Global1.vi" "联机模式"() -> (w663:enum16{"单机", "追溯"})
                    n281 = case shown="\"追溯\"" w663 {
                      selector: w663 -> [_ w673]
                      frame "单机", Default {
                      }
                      frame "追溯" {
                        n282 = shared-variable "我的电脑\\Global.lvlib\\传感器码-左"() -> (w664:string)  [unwired: 1 in, 1 out]
                        n283 = global read "追溯Global.vi" "PRODUCT_ID"() -> (w672:string)
                        n284 = Bundle("String"=w664, "PRODUCT_ID"=w672) -> (w670:cluster{"String":string, "PRODUCT_ID":string})  [unwired: 1 in]
                        n285 = call "GetSQLstring.vi"("联机模式"=w673) -> ("错误输出"=w669:errorcluster, "连接字符串"=w671:string)  [unwired: 9 in]
                        n286 = call-poly <vilib>:"DB Tools Open Connection.vi"("error in (no error)"=w669, "connection information"=w671) -> ("error out"=w666:errorcluster, "connection reference"=w668:T8)  [unwired: 6 in]
                        n287 = Build Array(w670) -> (w665:cluster{"String":string, "PRODUCT_ID":string}[])
                        n288 = for {
                          tunnel: w665 -> [w680] mode=indexing
                          tunnel: w668 -> [w679]
                          shift-right: [w675] -> w667
                          shift-left: w666 -> [w674]
                          n289 = call <vilib>:"DB Tools Insert Data.vi"("data"=w680, "error in (no error)"=w674, "columns"=string[] ["CODE_SENSOR", "PRODUCT_ID"], "table"="Code", "connection reference"=w679) -> ("error out"=w676:errorcluster)  [unwired: 5 in, 1 out]
                          n290 = case shown="无错误" w676 {
                            selector: w676 -> [w681 w682]
                            tunnel: [w681 w683] -> w675
                            frame No Error {
                            }
                            frame Error {
                              n291 = call <vilib>:"Clear Errors.vi"("error in (no error)"=w682) -> ("error out"=w683:errorcluster)  [unwired: 5 in, 1 out]
                            }
                          }
                        }
                        n292 = call <vilib>:"Simple Error Handler.vi"("error in (no error)"=w667) -> ()  [unwired: 4 in, 5 out]
                      }
                    }
                  }
                  frame #2 {
                    n293 = global read "Global1.vi" "联机模式"() -> (w684:enum16{"单机", "追溯"})
                    n294 = case shown="\"追溯\"" w684 {
                      selector: w684 -> [_ w705]
                      frame "单机", Default {
                      }
                      frame "追溯" {
                        w697 = "'"
                        n295 = shared-variable "我的电脑\\Global.lvlib\\传感器码-左"() -> (w685:string)  [unwired: 1 in, 1 out]
                        n296 = global read "追溯Global.vi" "PRODUCT_ID"() -> (w698:string)
                        n297 = call "GetSQLstring.vi"("联机模式"=w705) -> ("错误输出"=w703:errorcluster, "连接字符串"=w704:string)  [unwired: 9 in]
                        n298 = Concatenate Strings("SELECT CODE_ID FROM CODE  WHERE CODE_SENSOR = '" ("table"), w685, w697, " AND PRODUCT_ID='" ("字符串"), w698, w697) -> (w696:string)
                        n299 = call-poly <vilib>:"DB Tools Open Connection.vi"("error in (no error)"=w703, "connection information"=w704) -> ("error out"=w702:errorcluster, "connection reference"=w701:T8)  [unwired: 6 in]
                        n300 = call-poly <vilib>:"DB Tools Execute Query.vi"("error in (no error)"=w702, "SQL query"=w696, "connection reference"=w701) -> ("error out"=w695:errorcluster, "recordset reference"=w694:T9)  [unwired: 5 in]
                        n301 = call-poly <vilib>:"DB Tools Fetch Recordset Data.vi"("error in (no error)"=w695, "recordset reference"=w694) -> ("error out"=w693:errorcluster, "recordset data"=w692:variant[][])  [unwired: 3 in, 1 out]
                        n302 = Variant To Data(error in=w693, type=string[][] [], Variant=w692) -> (data=w690:string[][])  [unwired: 1 out]
                        n303 = Index Array(array=w690, index (row)=0 ("索引 (行)")) -> (element=w689:string[])  [unwired: 1 in]
                        n304 = Index Array(array=w689, index=0 ("索引")) -> (element=w688:string)
                        n305 = local write "左code"(w688) -> ()
                      }
                    }
                  }
                  frame #3 {
                    n306 = local write "STEP"("自动" ("STEP")) -> ()
                    n307 = call "左工位状态.vi"("枚举"=enum16{"Read", "Write"}."Write", "Status_Write"=u16 1003 ("左工位状态")) -> ()  [unwired: 9 in, 1 out]
                    n308 = for {
                      N: 12 -> [_]
                      tunnel: [cluster{dbl[], dbl[]} {[], []}] -> w712 mode=indexing
                    }
                    n309 = local write "左工位"(w712) -> ()
                    n310 = global read "Global.vi" "Result"() -> (w711:refnum<vi>)
                    n311 = property class="Tbl"(reference=w711, "Row Headers[]"=string[] [] ("行首字符串[]"), "Value"=string[][] [] ("值"), "Active Cell"=T2 {"Row"=-2, "Column"=-2} ("活动单元格:活动单元格"), "Cell BG Color"=u32 16777216 ("活动单元格:单元格背景色")) -> ()  [unwired: 1 in, 2 out]
                  }
                }
              }
            }
          }
          frame "不合格" {
            n312 = Wait (ms)(milliseconds to wait=u32 100 ("等待时间（毫秒）")) -> ()  [unwired: 1 out]
            n313 = local write "STEP"("等待" ("STEP")) -> ()
          }
          frame "报表" {
            n314 = global read "Global.vi" "左启用"() -> (w719:i16)
            n315 = case shown="1" w719 {
              frame 0, Default {
              }
              frame 1 {
                n316 = stacked-sequence {
                  frame #0 {
                    n317 = stacked-sequence {
                      seq-local: [w722 _ _] -> [_ w725 _]
                      frame #0 {
                        n318 = shared-variable "我的电脑\\Global.lvlib\\传感器码-左"() -> (w720:string)  [unwired: 1 in, 1 out]
                        n319 = call "Report.vi"("文件重命名"=TRUE, "文件名称"=w720, "检测结果"="判定结果") -> ("PRODUCT_VAULE"=w722:string)  [unwired: 7 in, 1 out]
                      }
                      frame #1 {
                        n320 = global read "Global1.vi" "联机模式"() -> (w724:enum16{"单机", "追溯"})
                        n321 = case shown="\"追溯\"" w724 {
                          tunnel: w725 -> [_ w729]
                          frame "单机", Default {
                          }
                          frame "追溯" {
                            n322 = global read "Global.vi" "Result"() -> (w733:refnum<vi>)
                            n323 = property class="Tbl"(reference=w733) -> (reference out=w732:refnum<vi>, "Row Headers[]"=w730:string[])  [unwired: 1 in, 1 out]
                            n324 = property class="Tbl"(reference=w732) -> ("Value"=w731:string[][])  [unwired: 1 in, 2 out]
                            n325 = for {
                              tunnel: w731 -> [w737] mode=indexing
                              tunnel: w730 -> [w738] mode=indexing
                              tunnel: [w735] -> w727 mode=indexing if=w736
                              n326 = Build Array (concatenate)(w738, w737) -> (w735:string[])
                              n327 = Index Array(array=w737) -> (element=w739:string)  [unwired: 1 in]
                              n328 = case shown="\"\"" w739 {
                                tunnel: [TRUE FALSE] -> w736
                                frame Default {
                                }
                                frame "" {
                                }
                              }
                            }
                            n329 = global read "追溯Global.vi" "DEVICE_ID"() -> (w728:string)
                            n330 = global read "追溯Global.vi" "USER_ID"() -> (w734:string)
                            n331 = local read "左code"() -> (w726:string)
                            n332 = call "UPTEST.vi"("Result"=w727, "CODE_ID"=w726, "DEVICE_ID"=w728) -> ()  [unwired: 6 in, 1 out]
                            n333 = call "UPRESULT.vi"("DEVICE_ID"=w728, "USER_ID"=w734, "CODE_ID"=w726, "RESULT_VALUE"=w729) -> ()  [unwired: 11 in, 1 out]
                          }
                        }
                      }
                      frame #2 {
                        n334 = Wait (ms)(milliseconds to wait=u32 50 ("等待时间（毫秒）")) -> ()  [unwired: 1 out]
                      }
                    }
                  }
                  frame #1 {
                    n335 = global write "Global.vi" "计时开始"(FALSE ("计时开始")) -> ()
                    n336 = call "左工位状态.vi"("枚举"=enum16{"Read", "Write"}."Write", "Status_Write"=i16 3) -> ()  [unwired: 9 in, 1 out]
                  }
                  frame #2 {
                    n337 = local write "STEP"("进入自动" ("STEP")) -> ()
                    n338 = global write "Global.vi" "计时开始"(FALSE ("计时开始")) -> ()
                  }
                }
              }
            }
          }
        }
        n339 = global read "Global.vi" "程序关闭"() -> (w374:bool)
        "STEP 4" <- "STEP"
      }
      n340 = while {
        stop <- w12 stop-if-true
        n341 = Wait (ms)(milliseconds to wait=u32 20 ("等待时间（毫秒）")) -> ()  [unwired: 1 out]
        n342 = case shown="\"报表\"" "STEP 2" {
          frame "等待", Default {
            n343 = Wait (ms)(milliseconds to wait=u32 200 ("等待时间（毫秒）")) -> ()  [unwired: 1 out]
            n344 = local write "STEP"("自动" ("STEP")) -> ()
          }
          frame "手动" {
          }
          frame "退出自动" {
            w16 = enum16{"Read", "Write"}."Write" ("枚举")
            n345 = global write "Global.vi" "计时开始"(FALSE ("计时开始")) -> ()
            n346 = local write "STEP 2"("等待" ("STEP")) -> ()
            n347 = call "设备状态.vi"("枚举"=w16, "Status_Write"=i16 0) -> ()  [unwired: 9 in, 1 out]
            n348 = call "跳转步骤.vi"("枚举"=w16, "Status_Write"=i16 1001) -> ()  [unwired: 9 in, 1 out]
          }
          frame "进入自动" {
            n349 = local write "STEP 2"("自动" ("STEP")) -> ()
            n350 = global read "Global.vi" "程序自动"() -> (w21:refnum<vi>)
            n351 = property class="Bool"(reference=w21, "Value"=TRUE) -> ()  [unwired: 1 in, 2 out]
          }
          frame "扫码" {
            n352 = stacked-sequence {
              frame #0 {
                w24 = "请扫传感器码！" ("提示信息")
                n353 = call "浮动通知.vi"("通知内容"=w24) -> ()  [unwired: 11 in]
                n354 = call "输入框.vi"("提示信息"=w24) -> ("条形码输出"=w25:string)
                n355 = case shown="\"\", \"exit\"" w25 {
                  selector: w25 -> [w26 _]
                  tunnel: [w28 "退出自动" ("State(s) in Front (\"\")")] -> w23
                  frame Default {
                    n356 = shared-variable "我的电脑\\Global.lvlib\\总成追溯码"(w26) -> ()  [unwired: 1 in, 1 out]
                    n357 = global read "Global1.vi" "联机模式"() -> (w27:enum16{"单机", "追溯"})
                    n358 = case shown="\"追溯\"" w27 {
                      tunnel: ["自动" ("State(s) in Front (\"\")") w34] -> w28
                      tunnel: w26 -> [_ w33]
                      frame "单机", Default {
                      }
                      frame "追溯" {
                        n359 = call "Get_CODE_ID.vi"("CODE_MAIN"=w33) -> ("CODE_ID"=w30:string)  [unwired: 10 in]
                        n360 = global write "追溯Global.vi" "CODE_ID 2"(w30) -> ()
                        n361 = global read "追溯Global.vi" "PRODUCT_ID"() -> (w32:string)
                        n362 = call "GET_PRESTATUS.vi"("CODE_ID"=w30, "PRODUCT_ID"=w32) -> ("OK?"=w31:bool)  [unwired: 8 in, 1 out]
                        n363 = case shown="假" w31 {
                          tunnel: [w38 "自动" ("State(s) in Front (\"\")")] -> w34
                          frame False {
                            n364 = global read "追溯Global.vi" "前序设备ID"() -> (w37:string)
                            n365 = Equal?(x=w37, y="") -> (x = y?=w36:bool)
                            n366 = case shown="真" w36 {
                              tunnel: ["退出自动" ("State(s) in Front (\"\")") "自动" ("State(s) in Front (\"\")")] -> w38
                              frame False {
                                n367 = global read "Global.vi" "上序状态"() -> (w41:refnum<vi>)
                                n368 = One Button Dialog(message="前序工位检测不合格！" ("消息")) -> ()  [unwired: 1 in, 1 out]
                                n369 = property class="Str"(reference=w41, "Text.BGColor"=u32 16711680 ("文本.文本颜色:背景色"), "Text.Text"="不合格" ("文本.文本")) -> ()  [unwired: 1 in, 2 out]
                              }
                              frame True {
                                n370 = global read "Global.vi" "上序状态"() -> (w46:refnum<vi>)
                                n371 = property class="Str"(reference=w46, "Text.BGColor"=u32 6618880 ("文本.文本颜色:背景色"), "Text.Text"="首序" ("文本.文本")) -> ()  [unwired: 1 in, 2 out]
                              }
                            }
                          }
                          frame True {
                            n372 = global read "Global.vi" "生产数量"() -> (w51:i32)
                            n373 = global read "Global.vi" "上序状态"() -> (w50:refnum<vi>)
                            n374 = Increment(x=w51) -> (x+1=w52:i32)
                            n375 = property class="Str"(reference=w50, "Text.BGColor"=u32 6618880 ("文本.文本颜色:背景色"), "Text.Text"="合格" ("文本.文本")) -> ()  [unwired: 1 in, 2 out]
                            n376 = global write "Global.vi" "生产数量"(w52) -> ()
                          }
                        }
                      }
                    }
                  }
                  frame "", "exit" {
                  }
                }
                n377 = local write "STEP 2"(w23) -> ()
              }
              frame #1 {
                n378 = Wait (ms)(milliseconds to wait=u32 200 ("等待时间（毫秒）")) -> ()  [unwired: 1 out]
              }
            }
          }
          frame "工位判断" {
          }
          frame "初始化" {
            n379 = stacked-sequence {
              frame #0 {
                n380 = for {
                  N: 12 -> [_]
                  tunnel: [cluster{dbl[], dbl[]} {[], []}] -> w57 mode=indexing
                }
                n381 = local write "判定结果 2"(bool[][] [] ("判定结果")) -> ()
                n382 = local write "右工位"(w57) -> ()
              }
              frame #1 {
                w60 = -2 ("维数大小")
                n383 = global read "Global.vi" "Result  右工位"() -> (w69:refnum<vi>)
                n384 = Initialize Array(TRUE, 12 ("维数大小")) -> (→"初始化 2":bool[])
                n385 = property class="Tbl"(reference=w69, "Value"=string[][] []) -> (reference out=w70:refnum<vi>, error out=w71:errorcluster)  [unwired: 1 in]
                n386 = property class="Tbl"(reference=w70, error in=w71, "Row Headers[]"=string[] [] ("列首字符串[]")) -> (reference out=w63:refnum<vi>)  [unwired: 1 out]
                n387 = Bundle("维数大小"=w60, "维数大小"=w60) -> (w61:cluster{"维数大小":i32, "维数大小":i32})  [unwired: 1 in]
                n388 = property class="Tbl"(reference=w63, "Active Cell"=w61, "Cell BG Color"=u32 16777216 ("活动单元格:单元格背景色")) -> ()  [unwired: 1 in, 2 out]
              }
              frame #2 {
                n389 = local write "STEP 2"("自动" ("STEP")) -> ()
              }
            }
          }
          frame "判定" {
            n390 = stacked-sequence {
              frame #0 {
                n391 = global read "Global.vi" "左启用"() -> (w73:i16)
                n392 = case shown="1" w73 {
                  tunnel: [w83 w84] -> w80
                  frame 0, Default {
                    n393 = global read "Global.vi" "Result"() -> (w83:refnum<vi>)
                  }
                  frame 1 {
                    n394 = global read "Global.vi" "Result  右工位"() -> (w84:refnum<vi>)
                  }
                }
                n395 = global read "A131258.vi" "结果判定参数"() -> (w78:T5)
                n396 = local read "右工位"() -> (w79:cluster{dbl[], dbl[]}[])
                n397 = call "试验判定 - 副本.vi"("Result"=w80, "判定参数"=w78, "XY曲线"=w79) -> ("判定项长度"=w77:i32, "OK？"=w81:bool)  [unwired: 7 in]
                n398 = local read "判定结果 2"() -> (w76:bool[][])
                n399 = case shown="真" w81 {
                  frame False {
                    n400 = call "右工位结果.vi"("枚举"=enum16{"Read", "Write"}."Write", "Status_Write"=u16 2 ("左工位生产结果")) -> ()  [unwired: 9 in, 1 out]
                  }
                  frame True {
                    n401 = call "右工位结果.vi"("枚举"=enum16{"Read", "Write"}."Write", "Status_Write"=u16 1 ("左工位生产结果")) -> ()  [unwired: 9 in, 1 out]
                  }
                }
                n402 = global write "判定参数.vi" "右判定长度"(w77) -> ()
                n403 = Build Array(TRUE ("元素"), w81) -> (w74:bool[])
                n404 = Build Array (concatenate)(w76, w74) -> (w75:bool[][])
                n405 = local write "判定结果 2"(w75) -> ()
              }
              frame #1 {
                n406 = local write "STEP 2"("报表" ("STEP")) -> ()
              }
            }
          }
          frame "自动" {
            n407 = global read "Global.vi" "右状态"() -> (w90:i16)
            n408 = case shown="1002" w90 {
              frame 0, Default {
              }
              frame 1 {
              }
              frame 3 {
                n409 = stacked-sequence {
                  frame #0 {
                    n410 = call "右工位结果.vi"("枚举"=enum16{"Read", "Write"}."Write", "Status_Write"=i16 0) -> ()  [unwired: 9 in, 1 out]
                    n411 = local write "判定结果 2"(bool[][] [] ("判定结果")) -> ()
                  }
                  frame #1 {
                    n412 = global read "Global.vi" "空载速度(°/s) 2"() -> (w94:sgl)
                    n413 = Multiply(x=w94, y=sgl 6.0) -> (x*y=w95:sgl)
                    n414 = global write "Global.vi" "空载速度(°/s)"(w95) -> ()
                  }
                }
              }
              frame 200 {
                n415 = stacked-sequence {
                  frame #0 {
                    w97 = TRUE ("Initialize 2")
                    n416 = local write "Initialize 7"(w97) -> ()
                    n417 = local write "Initialize 6"(w97) -> ()
                    n418 = call "右工位结果.vi"("枚举"=enum16{"Read", "Write"}."Write", "Status_Write"=u16 0 ("左工位生产结果")) -> ()  [unwired: 9 in, 1 out]
                  }
                  frame #1 {
                    n419 = local read "右工位"() -> (w100:cluster{dbl[], dbl[]}[])
                    n420 = for {
                      tunnel: [w103] -> w101 mode=indexing
                      tunnel: w100 -> [w102] mode=indexing
                      i -> [w104]
                      n421 = case shown="0" w104 {
                        tunnel: [w105 w106 w114] -> w103
                        tunnel: w102 -> [w105 _ _]
                        frame Default {
                        }
                        frame 0 {
                          n422 = global read "A131258.vi" "判定框参数"() -> (w111:T6)
                          n423 = Unbundle By Name(w111) -> ("正向判定X值.下限"=w110:dbl, "正向判定X值.上限"=w109:dbl, "正向判定Y值.下限"=w108:dbl, "正向判定Y值.上限"=w107:dbl)
                          n424 = Build Array(w109, w109, w110, w110, w109) -> (w113:dbl[])
                          n425 = Build Array(w107, w108, w108, w107, w107) -> (w112:dbl[])
                          n426 = Bundle(w113, w112) -> (w106:cluster{dbl[], dbl[]})  [unwired: 1 in]
                        }
                        frame 1 {
                          n427 = global read "A131258.vi" "判定框参数"() -> (w119:T6)
                          n428 = Unbundle By Name(w119) -> ("逆向判定X值.下限"=w118:dbl, "逆向判定X值.上限"=w117:dbl, "逆向判定Y值.下限"=w116:dbl, "逆向判定Y值.上限"=w115:dbl)
                          n429 = Build Array(w117, w117, w118, w118, w117) -> (w121:dbl[])
                          n430 = Build Array(w115, w116, w116, w115, w115) -> (w120:dbl[])
                          n431 = Bundle(w121, w120) -> (w114:cluster{dbl[], dbl[]})  [unwired: 1 in]
                        }
                      }
                    }
                    n432 = local write "右工位"(w101) -> ()
                  }
                }
              }
              frame 500 {
                n433 = local read "右工位"() -> (w123:cluster{dbl[], dbl[]}[])
                n434 = for {
                  tunnel: w123 -> [w125] mode=indexing
                  tunnel: [w124] -> w122 mode=indexing
                  i -> [w126]
                  n435 = case shown="2" w126 {
                    tunnel: w125 -> [w127 w144]
                    tunnel: [w127 w136] -> w124
                    frame Default {
                    }
                    frame 2 {
                      n436 = local write "Initialize 6"(FALSE ("Initialize 2")) -> ()
                      n437 = case shown="假" "Initialize 6" {
                        tunnel: [w157 0.0] -> w141
                        frame False {
                          n438 = global read "全局 1.vi" "工位1正向磨合开始时间"() -> (w161:u32)
                          n439 = Tick Count (ms)() -> (millisecond timer value=w160:u32)
                          n440 = Subtract(x=w160, y=w161) -> (x-y=w159:u32)
                          n441 = Divide(x=w159, y=u32 1000) -> (x/y=w157:dbl)
                          n442 = global write "全局 1.vi" "工位1正向磨合结束时间"(w157) -> ()
                        }
                        frame True {
                          n443 = Tick Count (ms)() -> (millisecond timer value=w162:u32)
                          n444 = global write "全局 1.vi" "工位1正向磨合开始时间"(w162) -> ()
                        }
                      }
                      n445 = global read "全局2.vi" "右加载"() -> (w129:dbl)
                      n446 = global read "A131258.vi" "零点标定"() -> (w131:bool)
                      n447 = global read "A131258.vi" "系数"() -> (w130:T7)
                      n448 = Unbundle(w144) -> (w138:dbl[], w143:dbl[])
                      n449 = case shown="假" w131 {
                        tunnel: [w146 w153] -> w128
                        tunnel: w130 -> [w152 w156]
                        tunnel: w129 -> [w151 w155]
                        frame False {
                          n450 = Unbundle By Name(w152) -> ("左零点漂移.正"=w150:dbl, "右空载.正转"=w147:dbl, "右零点漂移.正"=w145:dbl)
                          n451 = Multiply(x=w151, y=w150) -> (x*y=w148:dbl)
                          n452 = Subtract(x=w148, y=w147) -> (x-y=w149:dbl)
                          n453 = Subtract(x=w149, y=w145) -> (x-y=w146:dbl)
                        }
                        frame True {
                          n454 = Unbundle By Name(w156) -> ("右零点漂移.正"=w154:dbl)
                          n455 = Subtract(x=w155, y=w154) -> (x-y=w153:dbl)
                        }
                      }
                      n456 = Build Array (concatenate)(w143, w128) -> (w135:dbl[])
                      n457 = global read "Global.vi" "空载速度(°/s)"() -> (w140:sgl)
                      n458 = Divide(x=w141, y=1.0) -> (x/y=w133:dbl)
                      n459 = Multiply(x=w140, y=w133) -> (x*y=w139:dbl)
                      n460 = Build Array (concatenate)(w138, w139) -> (w137:dbl[])
                      n461 = Bundle(w137, w135) -> (w136:cluster{dbl[], dbl[]})  [unwired: 1 in]
                    }
                  }
                }
                n462 = local write "右工位"(w122) -> ()
              }
              frame 600 {
                n463 = local read "右工位"() -> (w165:cluster{dbl[], dbl[]}[])
                n464 = for {
                  tunnel: w165 -> [w167] mode=indexing
                  tunnel: [w166] -> w164 mode=indexing
                  i -> [w168]
                  n465 = case shown="3" w168 {
                    tunnel: w167 -> [w169 w186]
                    tunnel: [w169 w178] -> w166
                    frame 0, Default {
                    }
                    frame 3 {
                      n466 = local write "Initialize 7"(FALSE ("Initialize 2")) -> ()
                      n467 = case shown="假" "Initialize 7" {
                        tunnel: [w199 w206] -> w175
                        frame False {
                          n468 = global read "全局 1.vi" "工位1逆向磨合开始时间"() -> (w205:u32)
                          n469 = Tick Count (ms)() -> (millisecond timer value=w204:u32)
                          n470 = Subtract(x=w204, y=w205) -> (x-y=w203:u32)
                          n471 = global read "全局 1.vi" "工位1正向磨合结束时间"() -> (w201:dbl)
                          n472 = Divide(x=w203, y=u32 1000) -> (x/y=w200:dbl)
                          n473 = Subtract(x=w201, y=w200) -> (x-y=w199:dbl)
                        }
                        frame True {
                          n474 = Tick Count (ms)() -> (millisecond timer value=w207:u32)
                          n475 = global write "全局 1.vi" "工位1逆向磨合开始时间"(w207) -> ()
                          n476 = global read "全局 1.vi" "工位1正向磨合结束时间"() -> (w206:dbl)
                        }
                      }
                      n477 = global read "全局2.vi" "右加载"() -> (w171:dbl)
                      n478 = global read "A131258.vi" "系数"() -> (w172:T7)
                      n479 = Unbundle(w186) -> (w181:dbl[], w185:dbl[])
                      n480 = global read "A131258.vi" "零点标定"() -> (w173:bool)
                      n481 = case shown="假" w173 {
                        tunnel: [w188 w195] -> w170
                        tunnel: w172 -> [w194 w198]
                        tunnel: w171 -> [w193 w197]
                        frame False {
                          n482 = Unbundle By Name(w194) -> ("左零点漂移.反"=w192:dbl, "右空载.反转"=w189:dbl, "右零点漂移.反"=w187:dbl)
                          n483 = Multiply(x=w193, y=w192) -> (x*y=w190:dbl)
                          n484 = Subtract(x=w190, y=w189) -> (x-y=w191:dbl)
                          n485 = Subtract(x=w191, y=w187) -> (x-y=w188:dbl)
                        }
                        frame True {
                          n486 = Unbundle By Name(w198) -> ("右零点漂移.反"=w196:dbl)
                          n487 = Subtract(x=w197, y=w196) -> (x-y=w195:dbl)
                        }
                      }
                      n488 = Build Array (concatenate)(w185, w170) -> (w179:dbl[])
                      n489 = global read "Global.vi" "空载速度(°/s)"() -> (w183:sgl)
                      n490 = Divide(x=w175, y=1.0) -> (x/y=w176:dbl)
                      n491 = Multiply(x=w183, y=w176) -> (x*y=w182:dbl)
                      n492 = Build Array (concatenate)(w181, w182) -> (w180:dbl[])
                      n493 = Bundle(w180, w179) -> (w178:cluster{dbl[], dbl[]})  [unwired: 1 in]
                    }
                  }
                }
                n494 = local write "右工位"(w164) -> ()
              }
              frame 680 {
                n495 = stacked-sequence {
                  frame #0 {
                    n496 = Wait (ms)(milliseconds to wait=u32 5 ("等待时间（毫秒）")) -> ()  [unwired: 1 out]
                  }
                  frame #1 {
                    n497 = local write "STEP 2"("判定" ("STEP")) -> ()
                  }
                }
              }
              frame 730 {
              }
              frame 1001 {
                n498 = stacked-sequence {
                  frame #0 {
                    n499 = Wait (ms)(milliseconds to wait=u32 50 ("等待时间（毫秒）")) -> ()  [unwired: 1 out]
                    n500 = shared-variable "我的电脑\\Global.lvlib\\工位追溯码"() -> (w210:string)  [unwired: 1 in, 1 out]
                    n501 = shared-variable "我的电脑\\Global.lvlib\\传感器码-右"(w210) -> ()  [unwired: 1 in, 1 out]
                  }
                  frame #1 {
                    n502 = global read "Global1.vi" "联机模式"() -> (w212:enum16{"单机", "追溯"})
                    n503 = case shown="\"追溯\"" w212 {
                      selector: w212 -> [_ w222]
                      frame "单机", Default {
                      }
                      frame "追溯" {
                        n504 = shared-variable "我的电脑\\Global.lvlib\\传感器码-右"() -> (w213:string)  [unwired: 1 in, 1 out]
                        n505 = global read "追溯Global.vi" "PRODUCT_ID"() -> (w219:string)
                        n506 = Bundle("String"=w213, "PRODUCT_ID"=w219) -> (w218:cluster{"String":string, "PRODUCT_ID":string})  [unwired: 1 in]
                        n507 = call "GetSQLstring.vi"("联机模式"=w222) -> ("错误输出"=w220:errorcluster, "连接字符串"=w221:string)  [unwired: 9 in]
                        n508 = call-poly <vilib>:"DB Tools Open Connection.vi"("error in (no error)"=w220, "connection information"=w221) -> ("error out"=w216:errorcluster, "connection reference"=w217:T8)  [unwired: 6 in]
                        n509 = Build Array(w218) -> (w214:cluster{"String":string, "PRODUCT_ID":string}[])
                        n510 = for {
                          tunnel: w217 -> [w230]
                          shift-right: [w227] -> w215
                          shift-left: w216 -> [w229]
                          tunnel: w214 -> [w223] mode=indexing
                          n511 = call <vilib>:"DB Tools Insert Data.vi"("data"=w223, "error in (no error)"=w229, "columns"=string[] ["CODE_SENSOR", "PRODUCT_ID"], "table"="Code", "connection reference"=w230) -> ("error out"=w228:errorcluster, "connection reference out"=w226:T8)  [unwired: 5 in]
                          n512 = case shown="错误 .." w228 {
                            selector: w228 -> [w232 w234]
                            tunnel: [w232 w235] -> w227
                            tunnel: [w231 w233] -> _
                            tunnel: w226 -> [w231 w233]
                            frame No Error {
                            }
                            frame Error {
                              n513 = call <vilib>:"Clear Errors.vi"("error in (no error)"=w234) -> ("error out"=w235:errorcluster)  [unwired: 5 in, 1 out]
                            }
                          }
                        }
                        n514 = call <vilib>:"Simple Error Handler.vi"("error in (no error)"=w215) -> ()  [unwired: 4 in, 5 out]
                      }
                    }
                  }
                  frame #2 {
                    n515 = global read "Global1.vi" "联机模式"() -> (w236:enum16{"单机", "追溯"})
                    n516 = case shown="\"追溯\"" w236 {
                      selector: w236 -> [_ w257]
                      frame "单机", Default {
                      }
                      frame "追溯" {
                        w249 = "'"
                        n517 = shared-variable "我的电脑\\Global.lvlib\\传感器码-右"() -> (w237:string)  [unwired: 1 in, 1 out]
                        n518 = global read "追溯Global.vi" "PRODUCT_ID"() -> (w250:string)
                        n519 = call "GetSQLstring.vi"("联机模式"=w257) -> ("错误输出"=w255:errorcluster, "连接字符串"=w256:string)  [unwired: 9 in]
                        n520 = Concatenate Strings("SELECT CODE_ID FROM CODE  WHERE CODE_SENSOR = '" ("table"), w237, w249, " AND PRODUCT_ID='" ("字符串"), w250, w249) -> (w248:string)
                        n521 = call-poly <vilib>:"DB Tools Open Connection.vi"("error in (no error)"=w255, "connection information"=w256) -> ("error out"=w254:errorcluster, "connection reference"=w253:T8)  [unwired: 6 in]
                        n522 = call-poly <vilib>:"DB Tools Execute Query.vi"("error in (no error)"=w254, "SQL query"=w248, "connection reference"=w253) -> ("error out"=w247:errorcluster, "recordset reference"=w246:T9)  [unwired: 5 in]
                        n523 = call-poly <vilib>:"DB Tools Fetch Recordset Data.vi"("error in (no error)"=w247, "recordset reference"=w246) -> ("error out"=w245:errorcluster, "recordset data"=w244:variant[][])  [unwired: 3 in, 1 out]
                        n524 = Variant To Data(error in=w245, type=string[][] [], Variant=w244) -> (data=w242:string[][])  [unwired: 1 out]
                        n525 = Index Array(array=w242, index (row)=0 ("索引 (行)")) -> (element=w241:string[])  [unwired: 1 in]
                        n526 = Index Array(array=w241, index=0 ("索引")) -> (element=→"右code 2":string)
                      }
                    }
                  }
                  frame #3 {
                    n527 = Wait (ms)(milliseconds to wait=u32 50 ("等待时间（毫秒）")) -> ()  [unwired: 1 out]
                    n528 = local write "STEP 2"("自动" ("STEP")) -> ()
                    n529 = call "右工位状态.vi"("枚举"=enum16{"Read", "Write"}."Write", "Status_Write"=u16 1003 ("左工位状态")) -> ()  [unwired: 9 in, 1 out]
                    n530 = for {
                      N: 12 -> [_]
                      tunnel: [cluster{dbl[], dbl[]} {[], []}] -> w260 mode=indexing
                    }
                    n531 = local write "右工位"(w260) -> ()
                    n532 = global read "Global.vi" "左启用"() -> (w258:i16)
                    n533 = case shown="1" w258 {
                      frame 0, Default {
                        n534 = global read "Global.vi" "Result"() -> (w269:refnum<vi>)
                        n535 = property class="Tbl"(reference=w269, "Row Headers[]"=string[] [] ("行首字符串[]"), "Value"=string[][] [] ("值"), "Active Cell"=T2 {"Row"=-2, "Column"=-2} ("活动单元格:活动单元格"), "Cell BG Color"=u32 16777216 ("活动单元格:单元格背景色")) -> ()  [unwired: 1 in, 2 out]
                      }
                      frame 1 {
                        n536 = global read "Global.vi" "Result  右工位"() -> (w274:refnum<vi>)
                        n537 = property class="Tbl"(reference=w274, "Row Headers[]"=string[] [] ("行首字符串[]"), "Value"=string[][] [] ("值"), "Active Cell"=T2 {"Row"=-2, "Column"=-2} ("活动单元格:活动单元格"), "Cell BG Color"=u32 16777216 ("活动单元格:单元格背景色")) -> ()  [unwired: 1 in, 2 out]
                      }
                    }
                  }
                }
              }
              frame 1002 {
                n538 = stacked-sequence {
                  frame #0 {
                    n539 = Wait (ms)(milliseconds to wait=u32 100 ("等待时间（毫秒）")) -> ()  [unwired: 1 out]
                    n540 = shared-variable "我的电脑\\Global.lvlib\\总成追溯码"() -> (w276:string)  [unwired: 1 in, 1 out]
                    n541 = shared-variable "我的电脑\\Global.lvlib\\传感器码-右"(w276) -> ()  [unwired: 1 in, 1 out]
                  }
                  frame #1 {
                    n542 = global read "Global1.vi" "联机模式"() -> (w278:enum16{"单机", "追溯"})
                    n543 = case shown="\"追溯\"" w278 {
                      selector: w278 -> [_ w288]
                      frame "单机", Default {
                      }
                      frame "追溯" {
                        n544 = shared-variable "我的电脑\\Global.lvlib\\传感器码-右"() -> (w279:string)  [unwired: 1 in, 1 out]
                        n545 = global read "追溯Global.vi" "PRODUCT_ID"() -> (w287:string)
                        n546 = Bundle("String"=w279, "PRODUCT_ID"=w287) -> (w285:cluster{"String":string, "PRODUCT_ID":string})  [unwired: 1 in]
                        n547 = call "GetSQLstring.vi"("联机模式"=w288) -> ("错误输出"=w284:errorcluster, "连接字符串"=w286:string)  [unwired: 9 in]
                        n548 = call-poly <vilib>:"DB Tools Open Connection.vi"("error in (no error)"=w284, "connection information"=w286) -> ("error out"=w281:errorcluster, "connection reference"=w283:T8)  [unwired: 6 in]
                        n549 = Build Array(w285) -> (w280:cluster{"String":string, "PRODUCT_ID":string}[])
                        n550 = for {
                          tunnel: w280 -> [w295] mode=indexing
                          tunnel: w283 -> [w294]
                          shift-right: [w290] -> w282
                          shift-left: w281 -> [w289]
                          n551 = call <vilib>:"DB Tools Insert Data.vi"("data"=w295, "error in (no error)"=w289, "columns"=string[] ["CODE_SENSOR", "PRODUCT_ID"], "table"="Code", "connection reference"=w294) -> ("error out"=w291:errorcluster)  [unwired: 5 in, 1 out]
                          n552 = case shown="无错误" w291 {
                            selector: w291 -> [w296 w297]
                            tunnel: [w296 w298] -> w290
                            frame No Error {
                            }
                            frame Error {
                              n553 = call <vilib>:"Clear Errors.vi"("error in (no error)"=w297) -> ("error out"=w298:errorcluster)  [unwired: 5 in, 1 out]
                            }
                          }
                        }
                        n554 = call <vilib>:"Simple Error Handler.vi"("error in (no error)"=w282) -> ()  [unwired: 4 in, 5 out]
                      }
                    }
                  }
                  frame #2 {
                    n555 = global read "Global1.vi" "联机模式"() -> (w299:enum16{"单机", "追溯"})
                    n556 = case shown="\"追溯\"" w299 {
                      selector: w299 -> [_ w320]
                      frame "单机", Default {
                      }
                      frame "追溯" {
                        w312 = "'"
                        n557 = shared-variable "我的电脑\\Global.lvlib\\传感器码-右"() -> (w302:string)  [unwired: 1 in, 1 out]
                        n558 = global read "追溯Global.vi" "PRODUCT_ID"() -> (w313:string)
                        n559 = call "GetSQLstring.vi"("联机模式"=w320) -> ("错误输出"=w318:errorcluster, "连接字符串"=w319:string)  [unwired: 9 in]
                        n560 = Concatenate Strings("SELECT CODE_ID FROM CODE  WHERE CODE_SENSOR = '" ("table"), w302, w312, " AND PRODUCT_ID='" ("字符串"), w313, w312) -> (w311:string)
                        n561 = call-poly <vilib>:"DB Tools Open Connection.vi"("error in (no error)"=w318, "connection information"=w319) -> ("error out"=w317:errorcluster, "connection reference"=w316:T8)  [unwired: 6 in]
                        n562 = call-poly <vilib>:"DB Tools Execute Query.vi"("error in (no error)"=w317, "SQL query"=w311, "connection reference"=w316) -> ("error out"=w310:errorcluster, "recordset reference"=w309:T9)  [unwired: 5 in]
                        n563 = call-poly <vilib>:"DB Tools Fetch Recordset Data.vi"("error in (no error)"=w310, "recordset reference"=w309) -> ("error out"=w308:errorcluster, "recordset data"=w307:variant[][])  [unwired: 3 in, 1 out]
                        n564 = Variant To Data(error in=w308, type=string[][] [], Variant=w307) -> (data=w305:string[][])  [unwired: 1 out]
                        n565 = Index Array(array=w305, index (row)=0 ("索引 (行)")) -> (element=w304:string[])  [unwired: 1 in]
                        n566 = Index Array(array=w304, index=0 ("索引")) -> (element=w303:string)
                        n567 = local write "右code 2"(w303) -> ()
                      }
                    }
                  }
                  frame #3 {
                    n568 = Wait (ms)(milliseconds to wait=u32 50 ("等待时间（毫秒）")) -> ()  [unwired: 1 out]
                    n569 = local write "STEP 2"("自动" ("STEP 2")) -> ()
                    n570 = call "右工位状态.vi"("枚举"=enum16{"Read", "Write"}."Write", "Status_Write"=u16 1003 ("左工位状态")) -> ()  [unwired: 9 in, 1 out]
                    n571 = for {
                      N: 12 -> [_]
                      tunnel: [cluster{dbl[], dbl[]} {[], []}] -> w323 mode=indexing
                    }
                    n572 = local write "右工位"(w323) -> ()
                    n573 = global read "Global.vi" "左启用"() -> (w321:i16)
                    n574 = case shown="1" w321 {
                      frame 0, Default {
                        n575 = global read "Global.vi" "Result"() -> (w332:refnum<vi>)
                        n576 = property class="Tbl"(reference=w332, "Row Headers[]"=string[] [] ("行首字符串[]"), "Value"=string[][] [] ("值"), "Active Cell"=T2 {"Row"=-2, "Column"=-2} ("活动单元格:活动单元格"), "Cell BG Color"=u32 16777216 ("活动单元格:单元格背景色")) -> ()  [unwired: 1 in, 2 out]
                      }
                      frame 1 {
                        n577 = global read "Global.vi" "Result  右工位"() -> (w337:refnum<vi>)
                        n578 = property class="Tbl"(reference=w337, "Row Headers[]"=string[] [] ("行首字符串[]"), "Value"=string[][] [] ("值"), "Active Cell"=T2 {"Row"=-2, "Column"=-2} ("活动单元格:活动单元格"), "Cell BG Color"=u32 16777216 ("活动单元格:单元格背景色")) -> ()  [unwired: 1 in, 2 out]
                      }
                    }
                  }
                }
              }
            }
          }
          frame "不合格" {
            n579 = Wait (ms)(milliseconds to wait=u32 100 ("等待时间（毫秒）")) -> ()  [unwired: 1 out]
            n580 = local write "STEP 2"("等待" ("STEP")) -> ()
          }
          frame "报表" {
            n581 = stacked-sequence {
              frame #0 {
                n582 = stacked-sequence {
                  seq-local: [w343 _ _] -> [_ w346 _]
                  frame #0 {
                    n583 = shared-variable "我的电脑\\Global.lvlib\\传感器码-右"() -> (w342:string)  [unwired: 1 in, 1 out]
                    n584 = call "Report1.vi"("文件重命名"=TRUE, "文件名称"=w342, "检测结果"="判定结果 2") -> ("PRODUCT_VAULE"=w343:string)  [unwired: 7 in, 1 out]
                  }
                  frame #1 {
                    n585 = global read "Global1.vi" "联机模式"() -> (w345:enum16{"单机", "追溯"})
                    n586 = case shown="\"追溯\"" w345 {
                      tunnel: w346 -> [_ w348]
                      frame "单机", Default {
                      }
                      frame "追溯" {
                        n587 = global read "Global.vi" "左启用"() -> (w347:i16)
                        n588 = case shown="0, 默认" w347 {
                          tunnel: [w357 w358] -> w355
                          frame 0, Default {
                            n589 = global read "Global.vi" "Result"() -> (w357:refnum<vi>)
                          }
                          frame 1 {
                            n590 = global read "Global.vi" "Result  右工位"() -> (w358:refnum<vi>)
                          }
                        }
                        n591 = property class="Tbl"(reference=w355) -> (reference out=w354:refnum<vi>, "Row Headers[]"=w352:string[])  [unwired: 1 in, 1 out]
                        n592 = property class="Tbl"(reference=w354) -> ("Value"=w353:string[][])  [unwired: 1 in, 2 out]
                        n593 = for {
                          tunnel: w353 -> [w361] mode=indexing
                          tunnel: w352 -> [w362] mode=indexing
                          tunnel: [w359] -> w349 mode=indexing if=w360
                          n594 = Build Array (concatenate)(w362, w361) -> (w359:string[])
                          n595 = Index Array(array=w361) -> (element=w363:string)  [unwired: 1 in]
                          n596 = case shown="默认" w363 {
                            tunnel: [TRUE FALSE] -> w360
                            frame Default {
                            }
                            frame "" {
                            }
                          }
                        }
                        n597 = global read "追溯Global.vi" "DEVICE_ID"() -> (w351:string)
                        n598 = global read "追溯Global.vi" "USER_ID"() -> (w356:string)
                        n599 = local read "右code 2"() -> (w350:string)
                        n600 = call "UPRESULT - 副本.vi"("DEVICE_ID"=w351, "USER_ID"=w356, "CODE_ID"=w350, "RESULT_VALUE"=w348) -> ()  [unwired: 11 in, 1 out]
                        n601 = call "UPTEST - 副本.vi"("Result"=w349, "CODE_ID"=w350, "DEVICE_ID"=w351) -> ()  [unwired: 6 in, 1 out]
                      }
                    }
                  }
                  frame #2 {
                    n602 = local write "STEP 2"("自动" ("STEP 2")) -> ()
                  }
                }
              }
              frame #1 {
                n603 = global write "Global.vi" "计时开始"(FALSE ("计时开始")) -> ()
                n604 = call "右工位状态.vi"("枚举"=enum16{"Read", "Write"}."Write", "Status_Write"=i16 3) -> ()  [unwired: 9 in, 1 out]
              }
              frame #2 {
                n605 = local write "STEP"("进入自动" ("STEP")) -> ()
                n606 = global write "Global.vi" "计时开始"(FALSE ("计时开始")) -> ()
              }
            }
          }
        }
        n607 = global read "Global.vi" "程序关闭"() -> (w12:bool)
        "STEP 3" <- "STEP 2"
      }
    }
  }
